vi "FPGA_Check_Pins_target.vi"() -> ()   [LabVIEW 2018]
uses:
  <vilib>/Platform/TimedLoop/XDataNode/timing_clust.ctl
  <vilib>/Platform/TimedLoop/XDataNode/nitl_modes.ctl
  <vilib>/Platform/TimedLoop/XDataNode/wakeup.ctl
  <vilib>/rvi/Emulation/niFpgaGetClockAttributes.vi
  <vilib>/rvi/Emulation/niFpgaSctlEmulationGetInTimedLoop.vi
  <vilib>/rvi/Emulation/niFpgaEmulationReportErrorSimple.vi
  <vilib>/rvi/eio/common/nirviEmuTemplateMethod_errors.vi
  <vilib>/rvi/Emulation/niFpgaCriticalErrorInLSC.vi
  <vilib>/rvi/Emulation/niFpgaProcessEmulError.vi
  <vilib>/eio/EIONode/EIONode.xnode
  <vilib>/Platform/TimedLoop/XDataNode/XDataNode.xnode
  <vilib>/Platform/TimedLoop/XDataNode/XDNodeRunTimeDep.lvlib
panel:
  out "Delay B to A":i16
  out "0 (B to A)":bool
  out "1 (B to A)":bool
  out "2 (B to A)":bool
  out "3 (B to A)":bool
  out "4 (B to A)":bool
  out "5 (B to A)":bool
  out "6 (B to A)":bool
  out "7 (B to A)":bool
  out "DDCA_PFI1_Read (B to A)":bool
  out "DDCA_PFI2_Read (B to A)":bool
  out "DDCA_PFI3_Read (B to A)":bool
  out "Number (B to A)":i16
  out "Delay 0.0 (B to A)":i16
  out "Delay 0.1 (B to A)":i16
  out "Delay 0.2 (B to A)":i16
  out "Delay 0.3 (B to A)":i16
  out "Delay 0.4 (B to A)":i16
  out "Delay 0.5 (B to A)":i16
  out "Delay 0.6 (B to A)":i16
  out "Delay 0.7 (B to A)":i16
  out "Delay 1.0 (B to A)":i16
  out "Delay 1.1 (B to A)":i16
  out "Delay 1.2 (B to A)":i16
  out "Delay 1.3 (B to A)":i16
  out "Delay 1.4 (B to A)":i16
  out "Delay 1.5 (B to A)":i16
  out "Delay 1.6 (B to A)":i16
  out "Delay 1.7 (B to A)":i16
  out "Delay PFI1 (B to A)":i16
  out "Delay PFI2 (B to A)":i16
  out "Delay PFI3 (B to A)":i16
  out "Delay 2.0 (B to A)":i16
  out "Delay 2.1 (B to A)":i16
  out "Delay 2.2 (B to A)":i16
  out "Delay 2.3 (B to A)":i16
  out "Delay 2.4 (B to A)":i16
  out "Delay 2.5 (B to A)":i16
  out "Delay 2.6 (B to A)":i16
  out "Delay 2.7 (B to A)":i16
  out "Read Port 0 A":u8 format="%b"
  out "Read Port 1 A":u8 format="%b"
  out "Read Port 2 A":u8 format="%b"
  out "DDCA_PFI1_Read 3":bool
  out "DDCA_PFI2_Read 3":bool
  out "DDCA_PFI3_Read 3":bool
  out "Delay A to B":i16
  out "DDCB_PFI3_Read (A to B)":bool
  out "DDCB_PFI2_Read (A to B)":bool
  out "DDCB_PFI1_Read (A to B)":bool
  out "Read Port 2 B":u8 format="%b"
  out "Read Port 1 B":u8 format="%b"
  out "Read Port 0 B":u8 format="%b"
  out "Delay 2.0":i16
  out "Delay 2.1":i16
  out "Delay 2.2":i16
  out "Delay 2.3":i16
  out "Delay 2.4":i16
  out "Delay 2.5":i16
  out "Delay 2.6":i16
  out "Delay 2.7":i16
  out "Delay PFI1":i16
  out "Delay PFI2":i16
  out "Delay PFI3":i16
  out "Delay 1.0":i16
  out "Delay 1.1":i16
  out "Delay 1.2":i16
  out "Delay 1.3":i16
  out "Delay 1.4":i16
  out "Delay 1.5":i16
  out "Delay 1.6":i16
  out "Delay 1.7":i16
  out "Delay 0.7":i16
  out "Delay 0.6":i16
  out "Delay 0.5":i16
  out "Delay 0.4":i16
  out "Delay 0.3":i16
  out "Delay 0.2":i16
  out "Delay 0.1":i16
  out "PFI 3  (A to B)":bool
  out "PFI 2  (A to B)":bool
  out "PFI 1  (A to B)":bool
  out "7":bool
  out "6":bool
  out "5":bool
  out "4":bool
  out "3":bool
  out "2":bool
  out "1":bool
  out "0":bool
  in  "Counter":i16
  out "Delay 0.0":i16
  out "Operation compl":bool
  in  "Write to PFI":u8
  in  "Cycle":bool
  in  "A to B/B to A":bool
  in  "Write to":u8 format="%b"
  in  "Source Freq":refnum<k21>="100 MHz Clock"
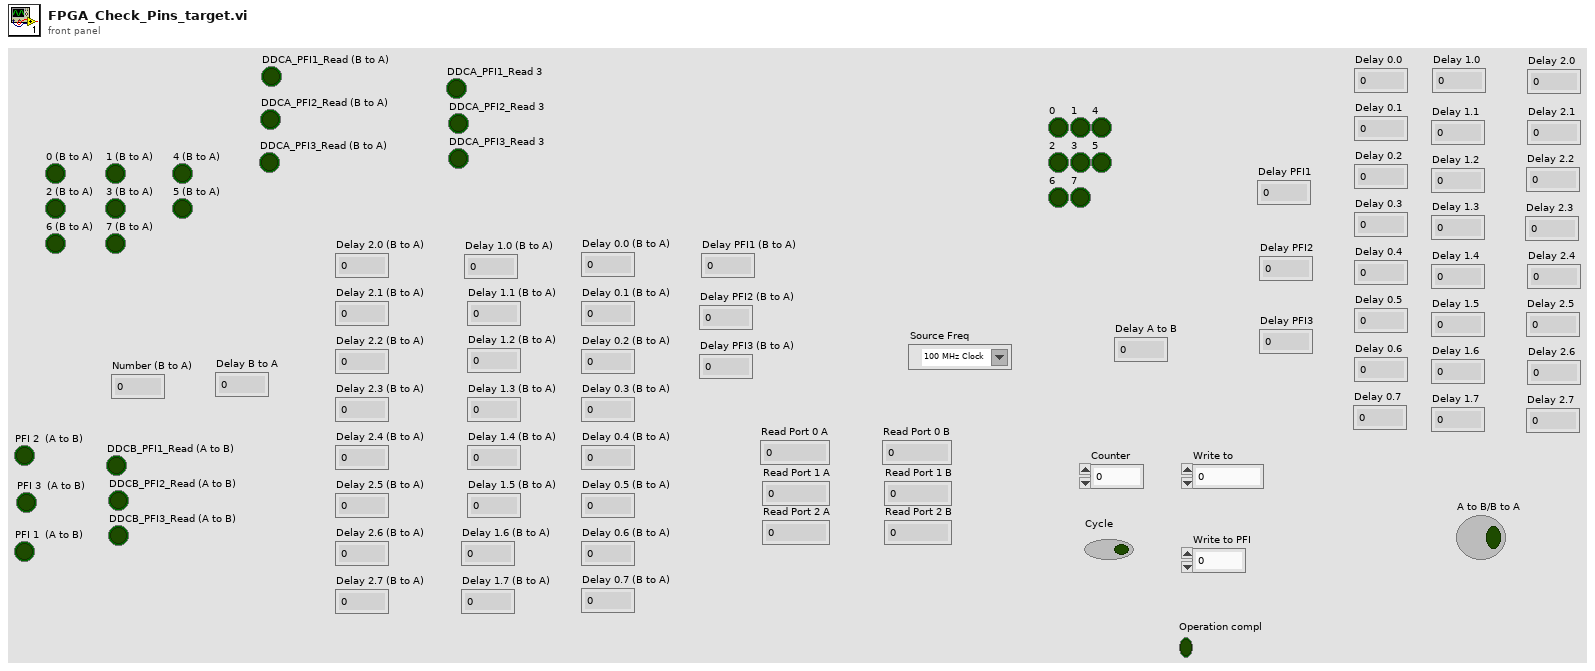
[diagram p1: front panel]
types:
  T1 = typedef "XDNodeRunTimeDep.lvlib/timing_clust.ctl" = cluster{"Expected End [f-1]":u64, "Actual End [f-1]":u64, "Finished Late? [f-1]":bool, "Expected End [i-1]":u64, "Actual End [i-1]":u64, "Finished Late? [i-1]":bool, "Expected Start [i]":u64, "Actual Start [i]":u64, "Expected Start [f]":u64, "Actual Start [f]":u64, "Source Name":string, "Structure Name":string, "Period":i64, "Deadline":i64, "Offset":i64, "Start":i64, "Priority":i32, "Timeout":i32, "Mode":T2, "Wakeup Reason":T3, "Error":errorcluster, "Source Type":string, "Secondary Source Type":string, "Global End Time":u64, "Global Start Time":u64, "Frame Duration":u64, "Iteration Duration":u64, "Assigned CPU":i32, "I/O Scan Engine Mode":u32}
  T2 = typedef "XDNodeRunTimeDep.lvlib/nitl_modes.ctl" = enum32{"No Change", "Process missed periods, maintain original phase", "Discard missed periods, maintain original phase", "Process missed periods, ignore original phase", "Discard missed periods, ignore original phase"}
  T3 = typedef "XDNodeRunTimeDep.lvlib/wakeup.ctl" = enum32{"Normal", "Aborted", "Asynchronous wakeup", "Timing source error", "Timed loop error", "Timeout"}
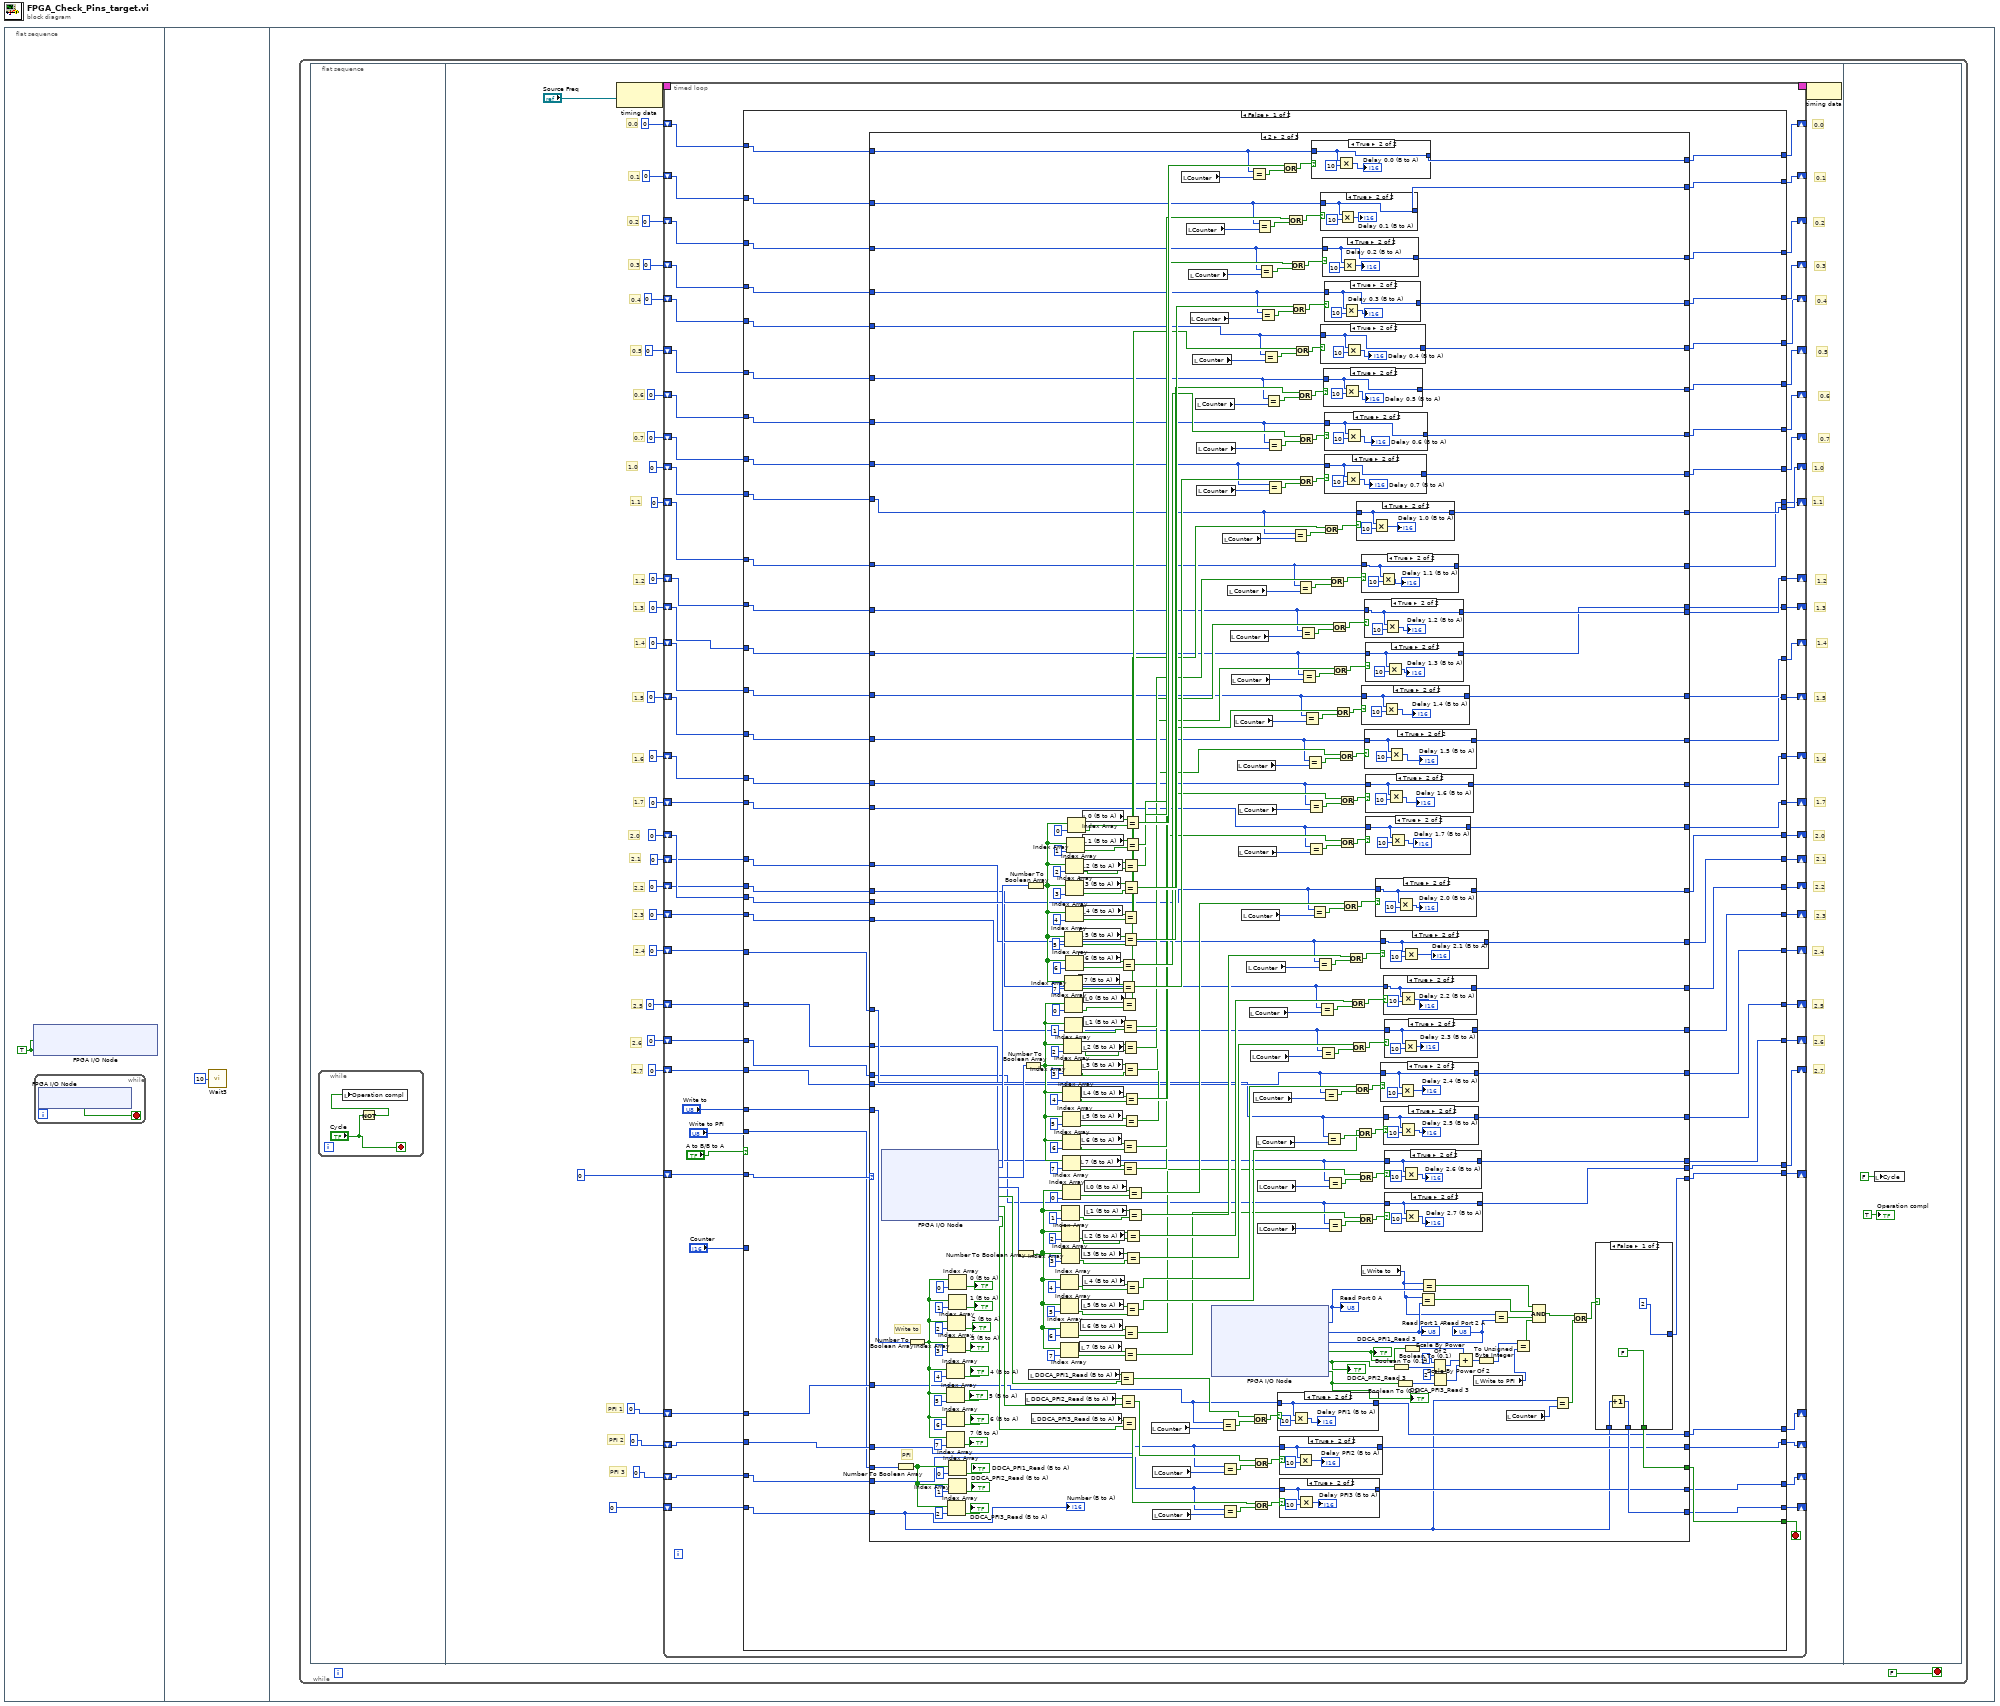
[diagram p0: block diagram]
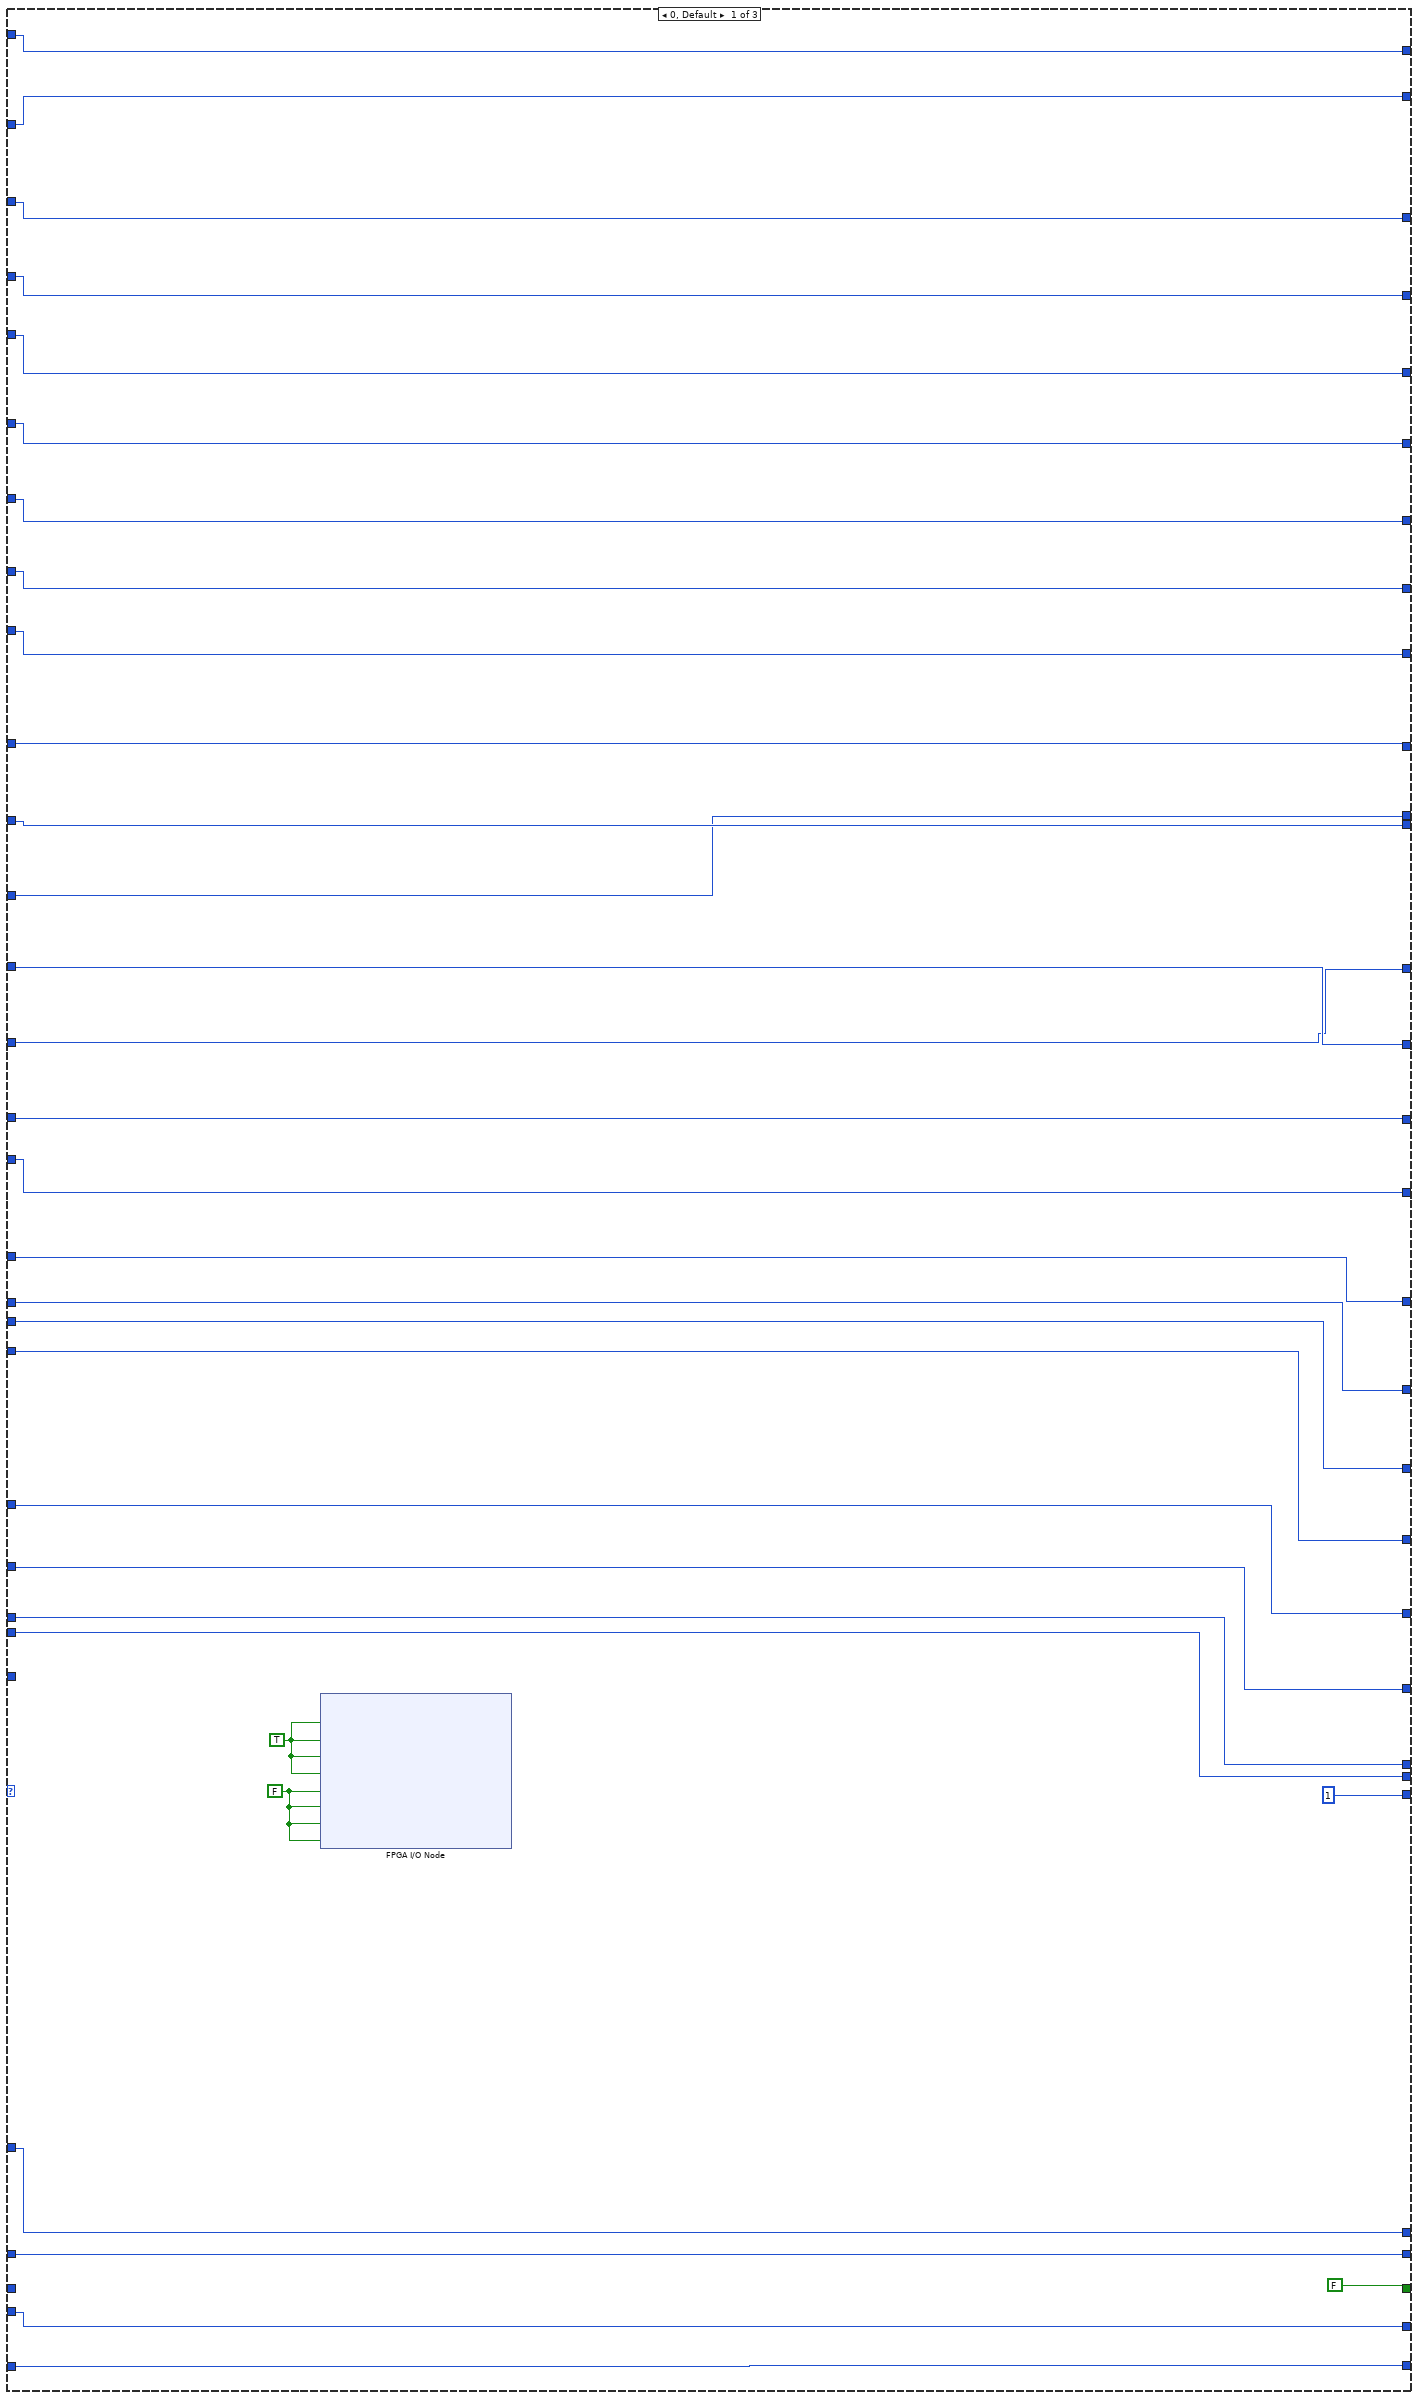
[diagram p2: hidden frame]
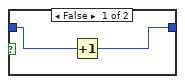
[diagram p3: hidden frame]
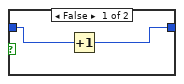
[diagram p4: hidden frame]
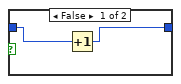
[diagram p5: hidden frame]
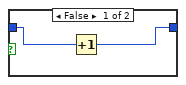
[diagram p6: hidden frame]
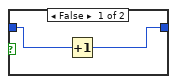
[diagram p7: hidden frame]
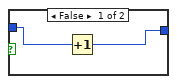
[diagram p8: hidden frame]
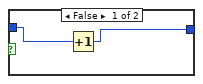
[diagram p9: hidden frame]
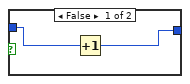
[diagram p10: hidden frame]
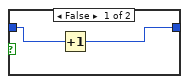
[diagram p11: hidden frame]
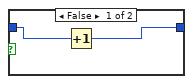
[diagram p12: hidden frame]
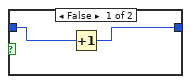
[diagram p13: hidden frame]
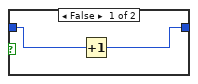
[diagram p14: hidden frame]
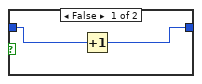
[diagram p15: hidden frame]
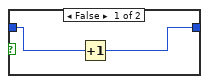
[diagram p16: hidden frame]
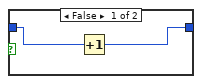
[diagram p17: hidden frame]
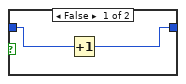
[diagram p18: hidden frame]
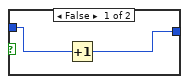
[diagram p19: hidden frame]
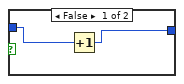
[diagram p20: hidden frame]
diagram:
  n1 = flat-sequence {
    frame #0 {
      w1 = TRUE ("IO Module\\DDCB_Supply_Select")
      n2 = xnode "FPGA I/O Node"("IO Module\\DDCB_Supply_Select"=w1, "IO Module\\DDCA_Supply_Select"=w1) -> ()  [unwired: 2 in, 2 out]
      n3 = while {
        stop <- w2 stop-if-true
        n4 = xnode "FPGA I/O Node"() -> ("IO Module IO Enabled"=w2:bool)  [unwired: 1 in, 1 out]
      }
    }
    frame #1 {
      n5 = call "Wait3"("Count(mSec)"=u8 10) -> ()  [unwired: 1 out]
    }
    frame #2 {
      n6 = while {
        stop <- FALSE stop-if-true
        n7 = flat-sequence {
          frame #0 {
            n8 = while {
              stop <- "Cycle" stop-if-true
              n9 = Not(x="Cycle") -> (.not. x?=w5:bool)
              n10 = local write "Operation compl"(w5) -> ()
            }
          }
          frame #1 {
            # "2.7"
            # "2.6"
            # "2.5"
            # "2.4"
            # "2.3"
            # "2.2"
            # "2.1"
            # "2.0"
            # "1.0"
            # "1.7"
            # "1.6"
            # "1.5"
            # "1.4"
            # "1.3"
            # "1.2"
            # "1.1"
            # "0.7"
            # "0.6"
            # "0.5"
            # "0.4"
            # "0.3"
            # "0.2"
            # "0.1"
            # "0.0"
            # "2.7"
            # "2.6"
            # "2.5"
            # "2.4"
            # "2.3"
            # "2.2"
            # "2.1"
            # "2.0"
            # "PFI 3"
            # "PFI 2"
            # "PFI 1"
            # "1.7"
            # "1.6"
            # "1.5"
            # "1.4"
            # "1.3"
            # "1.2"
            # "1.1"
            # "1.0"
            # "0.7"
            # "0.6"
            # "0.5"
            # "0.4"
            # "0.3"
            # "0.2"
            # "0.1"
            # "0.0"
            n11 = node-c288("Source Freq") -> (w38:T1)
            n12 = timed-loop {
              timing: w38 -> [_]
              timing-out: [_] -> w37
              shift-right: [w100] -> _
              shift-left: i16 0 -> [w101]
              shift-right: [w95] -> _
              shift-left: i16 0 -> [w94]
              shift-right: [w92] -> _
              shift-left: i16 0 -> [w91]
              shift-right: [w89] -> _
              shift-left: i16 0 -> [w90]
              shift-right: [w87] -> _
              shift-left: i16 0 -> [w88]
              shift-right: [w81] -> _
              shift-left: i16 0 -> [w86]
              shift-right: [w80] -> _
              shift-left: i16 0 -> [w85]
              shift-right: [w79] -> _
              shift-left: i16 0 -> [w84]
              shift-right: [w78] -> _
              shift-left: i16 0 -> [w83]
              shift-right: [w77] -> _
              shift-left: i16 0 -> [w82]
              shift-right: [w71] -> _
              shift-left: i16 0 -> [w76]
              shift-right: [w72] -> _
              shift-left: i16 0 -> [w75]
              shift-right: [w73] -> _
              shift-left: i16 0 -> [w74]
              shift-right: [w54] -> _
              shift-left: i16 0 -> [w70]
              shift-right: [w53] -> _
              shift-left: i16 0 -> [w69]
              shift-right: [w52] -> _
              shift-left: i16 0 -> [w68]
              shift-right: [w51] -> _
              shift-left: i16 0 -> [w67]
              shift-right: [w50] -> _
              shift-left: i16 0 -> [w66]
              shift-right: [w49] -> _
              shift-left: i16 0 -> [w65]
              shift-right: [w48] -> _
              shift-left: i16 0 -> [w64]
              shift-right: [w47] -> _
              shift-left: i16 0 -> [w63]
              shift-right: [w46] -> _
              shift-left: i16 0 -> [w62]
              shift-right: [w45] -> _
              shift-left: i16 0 -> [w61]
              shift-right: [w44] -> _
              shift-left: i16 0 -> [w60]
              shift-right: [w43] -> _
              shift-left: i16 0 -> [w59]
              shift-right: [w42] -> _
              shift-left: i16 0 -> [w58]
              shift-right: [w41] -> _
              shift-left: i16 0 -> [w57]
              shift-right: [w40] -> _
              shift-left: i16 0 -> [w56]
              shift-right: [w39] -> _
              shift-left: i16 0 -> [w55]
              stop <- w99 stop-if-true
              n13 = case shown="False" "A to B/B to A" {
                tunnel: w101 -> [w160 w738]
                tunnel: [w108 w737] -> w100
                tunnel: [w105 w736] -> w99
                tunnel: "Write to PFI" -> [w157 w678]
                tunnel: "Write to" -> [w156 w677]
                tunnel: [w104 w735] -> w95
                tunnel: w94 -> [w162 w734]
                tunnel: "Counter" -> [_ w733]
                tunnel: [w155 w732] -> w92
                tunnel: w91 -> [w154 w731]
                tunnel: w90 -> [w153 w730]
                tunnel: [w130 w729] -> w89
                tunnel: w88 -> [w152 w728]
                tunnel: [w129 w727] -> w87
                tunnel: w86 -> [w151 w726]
                tunnel: w85 -> [w150 w725]
                tunnel: w84 -> [w149 w724]
                tunnel: w83 -> [w148 w723]
                tunnel: w82 -> [w147 w722]
                tunnel: [w128 w721] -> w81
                tunnel: [w127 w720] -> w80
                tunnel: [w126 w719] -> w79
                tunnel: [w125 w718] -> w78
                tunnel: [w124 w717] -> w77
                tunnel: w76 -> [w159 w716]
                tunnel: w75 -> [w158 w715]
                tunnel: w74 -> [w161 w714]
                tunnel: [w103 w713] -> w73
                tunnel: [w102 w712] -> w72
                tunnel: [w106 w711] -> w71
                tunnel: w70 -> [w146 w710]
                tunnel: w69 -> [w145 w709]
                tunnel: w68 -> [w144 w708]
                tunnel: w67 -> [w143 w707]
                tunnel: w66 -> [w142 w706]
                tunnel: w65 -> [w141 w705]
                tunnel: w64 -> [w140 w704]
                tunnel: w63 -> [w139 w703]
                tunnel: w62 -> [w136 w702]
                tunnel: w61 -> [w138 w701]
                tunnel: w60 -> [w137 w700]
                tunnel: w59 -> [w135 w699]
                tunnel: w58 -> [w134 w698]
                tunnel: w57 -> [w133 w697]
                tunnel: w56 -> [w132 w696]
                tunnel: w55 -> [w131 w695]
                tunnel: [w123 w694] -> w54
                tunnel: [w122 w693] -> w53
                tunnel: [w121 w692] -> w52
                tunnel: [w120 w691] -> w51
                tunnel: [w119 w690] -> w50
                tunnel: [w118 w689] -> w49
                tunnel: [w117 w688] -> w48
                tunnel: [w116 w687] -> w47
                tunnel: [w115 w686] -> w46
                tunnel: [w114 w685] -> w45
                tunnel: [w113 w684] -> w44
                tunnel: [w112 w683] -> w43
                tunnel: [w111 w682] -> w42
                tunnel: [w110 w681] -> w41
                tunnel: [w109 w680] -> w40
                tunnel: [w107 w679] -> w39
                frame False {
                  n14 = case shown="2" w160 {
                    tunnel: [i16 1 w495 i16 2] -> w108
                    tunnel: [FALSE w494 FALSE] -> w105
                    tunnel: [w192 w249 w667] -> w104
                    tunnel: w162 -> [w192 w195 w667]
                    tunnel: w156 -> [_ w493 w638]
                    tunnel: w157 -> [_ w483 w639]
                    tunnel: [w189 w250 w666] -> w155
                    tunnel: w154 -> [w189 w248 w666]
                    tunnel: w153 -> [w188 w247 w665]
                    tunnel: [w188 w246 w665] -> w130
                    tunnel: w152 -> [w187 w245 w664]
                    tunnel: [w187 w244 w664] -> w129
                    tunnel: w151 -> [w186 w243 w663]
                    tunnel: w150 -> [w185 w242 w662]
                    tunnel: w149 -> [w184 w241 w661]
                    tunnel: w148 -> [w183 w240 w660]
                    tunnel: w147 -> [w182 w239 w659]
                    tunnel: [w186 w238 w663] -> w128
                    tunnel: [w185 w237 w662] -> w127
                    tunnel: [w184 w236 w661] -> w126
                    tunnel: [w183 w235 w660] -> w125
                    tunnel: [w182 w234 w659] -> w124
                    tunnel: w159 -> [w163 w233 w640]
                    tunnel: w158 -> [w164 w232 w641]
                    tunnel: w161 -> [w165 w231 w642]
                    tunnel: [w165 w230 w642] -> w103
                    tunnel: [w164 w229 w641] -> w102
                    tunnel: [w163 w228 w640] -> w106
                    tunnel: w146 -> [w181 w227 w658]
                    tunnel: w145 -> [w180 w226 w657]
                    tunnel: w144 -> [w179 w225 w656]
                    tunnel: w143 -> [w178 w224 w655]
                    tunnel: w142 -> [w177 w223 w654]
                    tunnel: w141 -> [w176 w222 w653]
                    tunnel: w140 -> [w175 w221 w652]
                    tunnel: w139 -> [w174 w220 w651]
                    tunnel: w136 -> [w171 w219 w650]
                    tunnel: w138 -> [w173 w218 w649]
                    tunnel: w137 -> [w172 w217 w648]
                    tunnel: w135 -> [w170 w216 w647]
                    tunnel: w131 -> [w166 w215 w643]
                    tunnel: w134 -> [w169 w214 w646]
                    tunnel: w133 -> [w168 w213 w645]
                    tunnel: w132 -> [w167 w212 w644]
                    tunnel: [w181 w211 w658] -> w123
                    tunnel: [w180 w210 w657] -> w122
                    tunnel: [w179 w209 w656] -> w121
                    tunnel: [w178 w208 w655] -> w120
                    tunnel: [w176 w207 w654] -> w119
                    tunnel: [w177 w206 w653] -> w118
                    tunnel: [w175 w205 w652] -> w117
                    tunnel: [w174 w204 w651] -> w116
                    tunnel: [w173 w203 w650] -> w115
                    tunnel: [w172 w202 w649] -> w114
                    tunnel: [w171 w201 w648] -> w113
                    tunnel: [w170 w200 w647] -> w112
                    tunnel: [w169 w199 w646] -> w111
                    tunnel: [w168 w198 w645] -> w110
                    tunnel: [w167 w197 w644] -> w109
                    tunnel: [w166 w196 w643] -> w107
                    frame 0, Default {
                      w190 = FALSE ("IO Module\\DDCB_Port0_WE")
                      w194 = TRUE
                      n15 = xnode "FPGA I/O Node"("IO Module\\DDCB_Port0_WE"=w194, "IO Module\\DDCB_Port1_WE"=w194, "IO Module\\DDCB_Port2_WE"=w194, "IO Module\\DDCB_PFI_WE"=w194, "IO Module\\DDCA_Port0_WE"=w190, "IO Module\\DDCA_Port1_WE"=w190, "IO Module\\DDCA_Port2_WE"=w190, "IO Module\\DDCA_PFI_WE"=w190) -> ()  [unwired: 8 in, 8 out]
                    }
                    frame 2 {
                      # "Write to"
                      # "PFI"
                      n16 = xnode "FPGA I/O Node"() -> ("IO Module\\DDCA_Port0_Read"=w469:u8, "IO Module\\DDCA_Port1_Read"=w459:u8, "IO Module\\DDCA_Port2_Read"=w449:u8, "IO Module\\DDCA_PFI1_Read"=w386:bool, "IO Module\\DDCA_PFI2_Read"=w385:bool, "IO Module\\DDCA_PFI3_Read"=w384:bool)  [unwired: 6 in, 6 out]
                      n17 = Number To Boolean Array(number=w483) -> (Boolean array=w479:bool[])
                      n18 = Number To Boolean Array(number=w493) -> (Boolean array=w492:bool[])
                      n19 = Index Array(array=w492, index=5) -> (element=→"5 (B to A)":bool)
                      n20 = Index Array(array=w492, index=7) -> (element=→"7 (B to A)":bool)
                      n21 = Index Array(array=w492, index=4) -> (element=→"4 (B to A)":bool)
                      n22 = Index Array(array=w492, index=6) -> (element=→"6 (B to A)":bool)
                      n23 = Index Array(array=w492, index=2) -> (element=→"2 (B to A)":bool)
                      n24 = Index Array(array=w492, index=3) -> (element=→"3 (B to A)":bool)
                      n25 = Index Array(array=w479, index=2) -> (element=→"DDCA_PFI3_Read (B to A)":bool)
                      n26 = Index Array(array=w492, index=1) -> (element=→"1 (B to A)":bool)
                      n27 = Index Array(array=w479, index=1) -> (element=→"DDCA_PFI2_Read (B to A)":bool)
                      n28 = Index Array(array=w492, index=0) -> (element=→"0 (B to A)":bool)
                      n29 = Index Array(array=w479, index=0) -> (element=→"DDCA_PFI1_Read (B to A)":bool)
                      n30 = Number To Boolean Array(number=w449) -> (Boolean array=w450:bool[])
                      n31 = Number To Boolean Array(number=w459) -> (Boolean array=w468:bool[])
                      n32 = local read "DDCA_PFI2_Read (B to A)"() -> (w388:bool)
                      n33 = Number To Boolean Array(number=w469) -> (Boolean array=w470:bool[])
                      n34 = local read "DDCA_PFI1_Read (B to A)"() -> (w389:bool)
                      n35 = local read "DDCA_PFI3_Read (B to A)"() -> (w387:bool)
                      n36 = Index Array(array=w450, index=5) -> (element=w392:bool)
                      n37 = Index Array(array=w450, index=7) -> (element=w390:bool)
                      n38 = Index Array(array=w450, index=4) -> (element=w393:bool)
                      n39 = Index Array(array=w450, index=6) -> (element=w391:bool)
                      n40 = Index Array(array=w450, index=2) -> (element=w395:bool)
                      n41 = Index Array(array=w450, index=3) -> (element=w394:bool)
                      n42 = Index Array(array=w450, index=1) -> (element=w396:bool)
                      n43 = Index Array(array=w468, index=5) -> (element=w408:bool)
                      n44 = Index Array(array=w468, index=7) -> (element=w406:bool)
                      n45 = Index Array(array=w450, index=0) -> (element=w397:bool)
                      n46 = Index Array(array=w468, index=4) -> (element=w409:bool)
                      n47 = Index Array(array=w468, index=6) -> (element=w407:bool)
                      n48 = Index Array(array=w468, index=2) -> (element=w411:bool)
                      n49 = Index Array(array=w468, index=3) -> (element=w410:bool)
                      n50 = Index Array(array=w468, index=1) -> (element=w412:bool)
                      n51 = Index Array(array=w470, index=5) -> (element=w426:bool)
                      n52 = Index Array(array=w470, index=7) -> (element=w422:bool)
                      n53 = Index Array(array=w468, index=0) -> (element=w413:bool)
                      n54 = Index Array(array=w470, index=4) -> (element=w428:bool)
                      n55 = Index Array(array=w470, index=6) -> (element=w424:bool)
                      n56 = Index Array(array=w470, index=2) -> (element=w432:bool)
                      n57 = Index Array(array=w470, index=3) -> (element=w430:bool)
                      n58 = Index Array(array=w470, index=1) -> (element=w434:bool)
                      n59 = Index Array(array=w470, index=0) -> (element=w437:bool)
                      n60 = local read "7 (B to A)"() -> (w423:bool)
                      n61 = local read "6 (B to A)"() -> (w425:bool)
                      n62 = local read "3 (B to A)"() -> (w431:bool)
                      n63 = local read "5 (B to A)"() -> (w427:bool)
                      n64 = local read "7 (B to A)"() -> (w421:bool)
                      n65 = local read "6 (B to A)"() -> (w420:bool)
                      n66 = local read "7 (B to A)"() -> (w398:bool)
                      n67 = local read "2 (B to A)"() -> (w433:bool)
                      n68 = local read "4 (B to A)"() -> (w429:bool)
                      n69 = local read "3 (B to A)"() -> (w417:bool)
                      n70 = local read "5 (B to A)"() -> (w419:bool)
                      n71 = local read "6 (B to A)"() -> (w399:bool)
                      n72 = local read "2 (B to A)"() -> (w416:bool)
                      n73 = local read "4 (B to A)"() -> (w418:bool)
                      n74 = local read "3 (B to A)"() -> (w402:bool)
                      n75 = local read "5 (B to A)"() -> (w400:bool)
                      n76 = local read "0 (B to A)"() -> (w436:bool)
                      n77 = local read "1 (B to A)"() -> (w435:bool)
                      n78 = local read "2 (B to A)"() -> (w403:bool)
                      n79 = local read "4 (B to A)"() -> (w401:bool)
                      n80 = local read "0 (B to A)"() -> (w414:bool)
                      n81 = local read "1 (B to A)"() -> (w415:bool)
                      n82 = local read "0 (B to A)"() -> (w405:bool)
                      n83 = local read "1 (B to A)"() -> (w404:bool)
                      n84 = Equal?(x=w389, y=w386) -> (x = y?=w309:bool)
                      n85 = Equal?(x=w388, y=w385) -> (x = y?=w308:bool)
                      n86 = Equal?(x=w425, y=w424) -> (x = y?=w353:bool)
                      n87 = Equal?(x=w423, y=w422) -> (x = y?=w352:bool)
                      n88 = Equal?(x=w414, y=w413) -> (x = y?=w326:bool)
                      n89 = Equal?(x=w387, y=w384) -> (x = y?=w307:bool)
                      n90 = Equal?(x=w415, y=w412) -> (x = y?=w325:bool)
                      n91 = Equal?(x=w420, y=w407) -> (x = y?=w320:bool)
                      n92 = Equal?(x=w421, y=w406) -> (x = y?=w319:bool)
                      n93 = Equal?(x=w429, y=w428) -> (x = y?=w364:bool)
                      n94 = Equal?(x=w427, y=w426) -> (x = y?=w354:bool)
                      n95 = Equal?(x=w416, y=w411) -> (x = y?=w324:bool)
                      n96 = Equal?(x=w398, y=w390) -> (x = y?=w275:bool)
                      n97 = Equal?(x=w433, y=w432) -> (x = y?=w372:bool)
                      n98 = Equal?(x=w431, y=w430) -> (x = y?=w368:bool)
                      n99 = Equal?(x=w417, y=w410) -> (x = y?=w323:bool)
                      n100 = Equal?(x=w399, y=w391) -> (x = y?=w276:bool)
                      n101 = Equal?(x=w418, y=w409) -> (x = y?=w322:bool)
                      n102 = Equal?(x=w419, y=w408) -> (x = y?=w321:bool)
                      n103 = Equal?(x=w436, y=w437) -> (x = y?=w383:bool)
                      n104 = Equal?(x=w435, y=w434) -> (x = y?=w376:bool)
                      n105 = Equal?(x=w401, y=w393) -> (x = y?=w278:bool)
                      n106 = Equal?(x=w400, y=w392) -> (x = y?=w277:bool)
                      n107 = Equal?(x=w403, y=w395) -> (x = y?=w280:bool)
                      n108 = Equal?(x=w402, y=w394) -> (x = y?=w279:bool)
                      n109 = Equal?(x=w405, y=w397) -> (x = y?=w282:bool)
                      n110 = Equal?(x=w404, y=w396) -> (x = y?=w281:bool)
                      n111 = local read "Counter"() -> (w316:i16)
                      n112 = local read "Counter"() -> (w315:i16)
                      n113 = local read "Counter"() -> (w310:i16)
                      n114 = local read "Counter"() -> (w382:i16)
                      n115 = local read "Counter"() -> (w377:i16)
                      n116 = local read "Counter"() -> (w375:i16)
                      n117 = local read "Counter"() -> (w369:i16)
                      n118 = local read "Counter"() -> (w367:i16)
                      n119 = local read "Counter"() -> (w361:i16)
                      n120 = local read "Counter"() -> (w360:i16)
                      n121 = local read "Counter"() -> (w355:i16)
                      n122 = xnode "FPGA I/O Node"() -> ("IO Module\\DDCA_Port0_Read"=w274:u8, "IO Module\\DDCA_Port1_Read"=w273:u8, "IO Module\\DDCA_Port2_Read"=w272:u8, "IO Module\\DDCA_PFI1_Read"=w271:bool, "IO Module\\DDCA_PFI2_Read"=w269:bool, "IO Module\\DDCA_PFI3_Read"=w270:bool)  [unwired: 6 in, 6 out]
                      "Read Port 0 A" <- w274
                      "Read Port 1 A" <- w273
                      "Read Port 2 A" <- w272
                      "DDCA_PFI1_Read 3" <- w271
                      "DDCA_PFI2_Read 3" <- w269
                      "DDCA_PFI3_Read 3" <- w270
                      n123 = Equal?(x=w233, y=w316) -> (x = y?=w317:bool)
                      n124 = Equal?(x=w232, y=w315) -> (x = y?=w314:bool)
                      n125 = Equal?(x=w231, y=w310) -> (x = y?=w311:bool)
                      n126 = local read "Counter"() -> (w327:i16)
                      n127 = local read "Counter"() -> (w332:i16)
                      n128 = local read "Counter"() -> (w333:i16)
                      n129 = local read "Counter"() -> (w338:i16)
                      n130 = local read "Counter"() -> (w339:i16)
                      n131 = local read "Counter"() -> (w344:i16)
                      n132 = local read "Counter"() -> (w345:i16)
                      n133 = local read "Counter"() -> (w350:i16)
                      n134 = local read "Counter"() -> (w306:i16)
                      n135 = local read "Counter"() -> (w301:i16)
                      n136 = local read "Counter"() -> (w300:i16)
                      n137 = Equal?(x=w248, y=w382) -> (x = y?=w381:bool)
                      n138 = local read "Counter"() -> (w295:i16)
                      n139 = Or(x=w309, y=w317) -> (x .or. y?=w318:bool)
                      n140 = Or(x=w308, y=w314) -> (x .or. y?=w313:bool)
                      n141 = Or(x=w307, y=w311) -> (x .or. y?=w312:bool)
                      n142 = local read "Counter"() -> (w294:i16)
                      n143 = Equal?(x=w247, y=w377) -> (x = y?=w378:bool)
                      n144 = local read "Counter"() -> (w289:i16)
                      n145 = local read "Counter"() -> (w288:i16)
                      n146 = local read "Counter"() -> (w283:i16)
                      n147 = Equal?(x=w245, y=w375) -> (x = y?=w374:bool)
                      n148 = Equal?(x=w243, y=w369) -> (x = y?=w370:bool)
                      n149 = Equal?(x=w242, y=w367) -> (x = y?=w366:bool)
                      n150 = Equal?(x=w241, y=w361) -> (x = y?=w362:bool)
                      n151 = Equal?(x=w240, y=w360) -> (x = y?=w359:bool)
                      n152 = Equal?(x=w239, y=w355) -> (x = y?=w356:bool)
                      n153 = case shown="True" w318 {
                        tunnel: w233 -> [w547 w548]
                        tunnel: [w546 w548] -> w228
                        frame False {
                          n154 = Increment(x=w547) -> (x+1=w546:i16)
                        }
                        frame True {
                          n155 = Multiply(x=w548, y=i16 10) -> (x*y=→"Delay PFI1 (B to A)":i16)
                        }
                      }
                      n156 = case shown="True" w313 {
                        tunnel: w232 -> [w542 w544]
                        tunnel: [w541 w544] -> w229
                        frame False {
                          n157 = Increment(x=w542) -> (x+1=w541:i16)
                        }
                        frame True {
                          n158 = Multiply(x=w544, y=i16 10) -> (x*y=→"Delay PFI2 (B to A)":i16)
                        }
                      }
                      n159 = case shown="True" w312 {
                        tunnel: w231 -> [w537 w539]
                        tunnel: [w536 w539] -> w230
                        frame False {
                          n160 = Increment(x=w537) -> (x+1=w536:i16)
                        }
                        frame True {
                          n161 = Multiply(x=w539, y=i16 10) -> (x*y=→"Delay PFI3 (B to A)":i16)
                        }
                      }
                      n162 = Or(x=w383, y=w381) -> (x .or. y?=w380:bool)
                      n163 = Or(x=w376, y=w378) -> (x .or. y?=w379:bool)
                      n164 = Or(x=w372, y=w374) -> (x .or. y?=w373:bool)
                      n165 = Or(x=w368, y=w370) -> (x .or. y?=w371:bool)
                      n166 = Equal?(x=w227, y=w327) -> (x = y?=w328:bool)
                      n167 = Or(x=w364, y=w366) -> (x .or. y?=w365:bool)
                      n168 = Or(x=w354, y=w362) -> (x .or. y?=w363:bool)
                      n169 = Equal?(x=w226, y=w332) -> (x = y?=w331:bool)
                      n170 = Or(x=w353, y=w359) -> (x .or. y?=w358:bool)
                      n171 = Or(x=w352, y=w356) -> (x .or. y?=w357:bool)
                      n172 = Equal?(x=w225, y=w333) -> (x = y?=w334:bool)
                      n173 = Equal?(x=w224, y=w338) -> (x = y?=w337:bool)
                      n174 = Equal?(x=w223, y=w339) -> (x = y?=w340:bool)
                      n175 = Equal?(x=w222, y=w344) -> (x = y?=w343:bool)
                      n176 = Equal?(x=w221, y=w345) -> (x = y?=w346:bool)
                      n177 = Equal?(x=w220, y=w350) -> (x = y?=w349:bool)
                      n178 = Equal?(x=w219, y=w306) -> (x = y?=w305:bool)
                      n179 = case shown="True" w380 {
                        tunnel: w248 -> [w626 w630]
                        tunnel: [w627 w630] -> w250
                        frame False {
                          n180 = Increment(x=w626) -> (x+1=w627:i16)
                        }
                        frame True {
                          n181 = Multiply(x=w630, y=i16 10) -> (x*y=→"Delay 0.0 (B to A)":i16)
                        }
                      }
                      n182 = Equal?(x=w218, y=w301) -> (x = y?=w302:bool)
                      n183 = Equal?(x=w217, y=w300) -> (x = y?=w299:bool)
                      n184 = Equal?(x=w216, y=w295) -> (x = y?=w296:bool)
                      n185 = case shown="True" w379 {
                        tunnel: w247 -> [w622 w623]
                        tunnel: [w621 w623] -> w246
                        frame False {
                          n186 = Increment(x=w622) -> (x+1=w621:i16)
                        }
                        frame True {
                          n187 = Multiply(x=w623, y=i16 10) -> (x*y=→"Delay 0.1 (B to A)":i16)
                        }
                      }
                      n188 = case shown="True" w365 {
                        tunnel: w242 -> [w607 w609]
                        tunnel: [w606 w609] -> w237
                        frame False {
                          n189 = Increment(x=w607) -> (x+1=w606:i16)
                        }
                        frame True {
                          n190 = Multiply(x=w609, y=i16 10) -> (x*y=→"Delay 0.4 (B to A)":i16)
                        }
                      }
                      n191 = Equal?(x=w215, y=w294) -> (x = y?=w293:bool)
                      n192 = case shown="True" w373 {
                        tunnel: w245 -> [w617 w619]
                        tunnel: [w616 w619] -> w244
                        frame False {
                          n193 = Increment(x=w617) -> (x+1=w616:i16)
                        }
                        frame True {
                          n194 = Multiply(x=w619, y=i16 10) -> (x*y=→"Delay 0.2 (B to A)":i16)
                        }
                      }
                      n195 = Or(x=w326, y=w328) -> (x .or. y?=w329:bool)
                      n196 = case shown="True" w363 {
                        tunnel: w241 -> [w602 w603]
                        tunnel: [w601 w603] -> w236
                        frame False {
                          n197 = Increment(x=w602) -> (x+1=w601:i16)
                        }
                        frame True {
                          n198 = Multiply(x=w603, y=i16 10) -> (x*y=→"Delay 0.5 (B to A)":i16)
                        }
                      }
                      n199 = case shown="True" w371 {
                        tunnel: w243 -> [w612 w613]
                        tunnel: [w611 w613] -> w238
                        frame False {
                          n200 = Increment(x=w612) -> (x+1=w611:i16)
                        }
                        frame True {
                          n201 = Multiply(x=w613, y=i16 10) -> (x*y=→"Delay 0.3 (B to A)":i16)
                        }
                      }
                      n202 = case shown="True" w358 {
                        tunnel: w240 -> [w597 w599]
                        tunnel: [w596 w599] -> w235
                        frame False {
                          n203 = Increment(x=w597) -> (x+1=w596:i16)
                        }
                        frame True {
                          n204 = Multiply(x=w599, y=i16 10) -> (x*y=→"Delay 0.6 (B to A)":i16)
                        }
                      }
                      n205 = case shown="True" w357 {
                        tunnel: w239 -> [w592 w593]
                        tunnel: [w591 w593] -> w234
                        frame False {
                          n206 = Increment(x=w592) -> (x+1=w591:i16)
                        }
                        frame True {
                          n207 = Multiply(x=w593, y=i16 10) -> (x*y=→"Delay 0.7 (B to A)":i16)
                        }
                      }
                      n208 = Equal?(x=w214, y=w289) -> (x = y?=w290:bool)
                      n209 = Equal?(x=w213, y=w288) -> (x = y?=w287:bool)
                      n210 = Equal?(x=w212, y=w283) -> (x = y?=w284:bool)
                      n211 = Or(x=w325, y=w331) -> (x .or. y?=w330:bool)
                      n212 = Or(x=w324, y=w334) -> (x .or. y?=w335:bool)
                      n213 = Or(x=w323, y=w337) -> (x .or. y?=w336:bool)
                      n214 = Or(x=w322, y=w340) -> (x .or. y?=w341:bool)
                      n215 = Or(x=w321, y=w343) -> (x .or. y?=w342:bool)
                      n216 = Or(x=w320, y=w346) -> (x .or. y?=w347:bool)
                      n217 = Or(x=w319, y=w349) -> (x .or. y?=w348:bool)
                      n218 = Or(x=w282, y=w305) -> (x .or. y?=w304:bool)
                      n219 = Or(x=w281, y=w302) -> (x .or. y?=w303:bool)
                      n220 = Or(x=w280, y=w299) -> (x .or. y?=w298:bool)
                      n221 = Or(x=w279, y=w296) -> (x .or. y?=w297:bool)
                      n222 = Or(x=w278, y=w293) -> (x .or. y?=w292:bool)
                      n223 = case shown="True" w329 {
                        tunnel: w227 -> [w587 w589]
                        tunnel: [w586 w589] -> w211
                        frame False {
                          n224 = Increment(x=w587) -> (x+1=w586:i16)
                        }
                        frame True {
                          n225 = Multiply(x=w589, y=i16 10) -> (x*y=→"Delay 1.0 (B to A)":i16)
                        }
                      }
                      n226 = Or(x=w277, y=w290) -> (x .or. y?=w291:bool)
                      n227 = Or(x=w276, y=w287) -> (x .or. y?=w286:bool)
                      n228 = Or(x=w275, y=w284) -> (x .or. y?=w285:bool)
                      n229 = local read "Write to"() -> (w260:u8)
                      n230 = case shown="True" w330 {
                        tunnel: w226 -> [w582 w584]
                        tunnel: [w581 w584] -> w210
                        frame False {
                          n231 = Increment(x=w582) -> (x+1=w581:i16)
                        }
                        frame True {
                          n232 = Multiply(x=w584, y=i16 10) -> (x*y=→"Delay 1.1 (B to A)":i16)
                        }
                      }
                      n233 = case shown="True" w341 {
                        tunnel: w223 -> [w567 w569]
                        tunnel: [w566 w569] -> w207
                        frame False {
                          n234 = Increment(x=w567) -> (x+1=w566:i16)
                        }
                        frame True {
                          n235 = Multiply(x=w569, y=i16 10) -> (x*y=→"Delay 1.4 (B to A)":i16)
                        }
                      }
                      n236 = case shown="True" w335 {
                        tunnel: w225 -> [w577 w578]
                        tunnel: [w576 w578] -> w209
                        frame False {
                          n237 = Increment(x=w577) -> (x+1=w576:i16)
                        }
                        frame True {
                          n238 = Multiply(x=w578, y=i16 10) -> (x*y=→"Delay 1.2 (B to A)":i16)
                        }
                      }
                      n239 = case shown="True" w342 {
                        tunnel: w222 -> [w562 w564]
                        tunnel: [w561 w564] -> w206
                        frame False {
                          n240 = Increment(x=w562) -> (x+1=w561:i16)
                        }
                        frame True {
                          n241 = Multiply(x=w564, y=i16 10) -> (x*y=→"Delay 1.5 (B to A)":i16)
                        }
                      }
                      n242 = case shown="True" w336 {
                        tunnel: w224 -> [w572 w573]
                        tunnel: [w571 w573] -> w208
                        frame False {
                          n243 = Increment(x=w572) -> (x+1=w571:i16)
                        }
                        frame True {
                          n244 = Multiply(x=w573, y=i16 10) -> (x*y=→"Delay 1.3 (B to A)":i16)
                        }
                      }
                      n245 = case shown="True" w347 {
                        tunnel: w221 -> [w557 w558]
                        tunnel: [w556 w558] -> w205
                        frame False {
                          n246 = Increment(x=w557) -> (x+1=w556:i16)
                        }
                        frame True {
                          n247 = Multiply(x=w558, y=i16 10) -> (x*y=→"Delay 1.6 (B to A)":i16)
                        }
                      }
                      n248 = case shown="True" w348 {
                        tunnel: w220 -> [w552 w553]
                        tunnel: [w551 w553] -> w204
                        frame False {
                          n249 = Increment(x=w552) -> (x+1=w551:i16)
                        }
                        frame True {
                          n250 = Multiply(x=w553, y=i16 10) -> (x*y=→"Delay 1.7 (B to A)":i16)
                        }
                      }
                      n251 = case shown="True" w304 {
                        tunnel: w219 -> [w532 w533]
                        tunnel: [w531 w533] -> w203
                        frame False {
                          n252 = Increment(x=w532) -> (x+1=w531:i16)
                        }
                        frame True {
                          n253 = Multiply(x=w533, y=i16 10) -> (x*y=→"Delay 2.0 (B to A)":i16)
                        }
                      }
                      n254 = case shown="True" w303 {
                        tunnel: w218 -> [w527 w529]
                        tunnel: [w526 w529] -> w202
                        frame False {
                          n255 = Increment(x=w527) -> (x+1=w526:i16)
                        }
                        frame True {
                          n256 = Multiply(x=w529, y=i16 10) -> (x*y=→"Delay 2.1 (B to A)":i16)
                        }
                      }
                      n257 = case shown="True" w292 {
                        tunnel: w215 -> [w512 w514]
                        tunnel: [w511 w514] -> w199
                        frame False {
                          n258 = Increment(x=w512) -> (x+1=w511:i16)
                        }
                        frame True {
                          n259 = Multiply(x=w514, y=i16 10) -> (x*y=→"Delay 2.4 (B to A)":i16)
                        }
                      }
                      n260 = case shown="True" w298 {
                        tunnel: w217 -> [w522 w523]
                        tunnel: [w521 w523] -> w201
                        frame False {
                          n261 = Increment(x=w522) -> (x+1=w521:i16)
                        }
                        frame True {
                          n262 = Multiply(x=w523, y=i16 10) -> (x*y=→"Delay 2.2 (B to A)":i16)
                        }
                      }
                      n263 = case shown="True" w291 {
                        tunnel: w214 -> [w507 w509]
                        tunnel: [w506 w509] -> w198
                        frame False {
                          n264 = Increment(x=w507) -> (x+1=w506:i16)
                        }
                        frame True {
                          n265 = Multiply(x=w509, y=i16 10) -> (x*y=→"Delay 2.5 (B to A)":i16)
                        }
                      }
                      n266 = case shown="True" w297 {
                        tunnel: w216 -> [w517 w519]
                        tunnel: [w516 w519] -> w200
                        frame False {
                          n267 = Increment(x=w517) -> (x+1=w516:i16)
                        }
                        frame True {
                          n268 = Multiply(x=w519, y=i16 10) -> (x*y=→"Delay 2.3 (B to A)":i16)
                        }
                      }
                      n269 = case shown="True" w286 {
                        tunnel: w213 -> [w502 w504]
                        tunnel: [w501 w504] -> w197
                        frame False {
                          n270 = Increment(x=w502) -> (x+1=w501:i16)
                        }
                        frame True {
                          n271 = Multiply(x=w504, y=i16 10) -> (x*y=→"Delay 2.6 (B to A)":i16)
                        }
                      }
                      n272 = case shown="True" w285 {
                        tunnel: w212 -> [w497 w499]
                        tunnel: [w496 w499] -> w196
                        frame False {
                          n273 = Increment(x=w497) -> (x+1=w496:i16)
                        }
                        frame True {
                          n274 = Multiply(x=w499, y=i16 10) -> (x*y=→"Delay 2.7 (B to A)":i16)
                        }
                      }
                      n275 = Boolean To (0,1)(Boolean=w269) -> (0, 1=w267:i16)
                      n276 = Boolean To (0,1)(Boolean=w270) -> (0, 1=w264:i16)
                      n277 = Boolean To (0,1)(Boolean=w271) -> (0, 1=w268:i16)
                      n278 = Equal?(x=w260, y=w273) -> (x = y?=w258:bool)
                      n279 = Equal?(x=w260, y=w274) -> (x = y?=w259:bool)
                      n280 = Scale By Power Of 2(n=i16 1, x=w267) -> (x*2^n=w265:i16)
                      n281 = Scale By Power Of 2(n=i16 2, x=w264) -> (x*2^n=w262:i16)
                      n282 = Compound Arithmetic op=unknown(w268, w265, w262) -> (w261:i16)
                      n283 = local read "Write to PFI"() -> (w251:u8)
                      n284 = To Unsigned Byte Integer(number=w261) -> (unsigned 8bit integer=w252:u8)
                      n285 = Equal?(x=w260, y=w272) -> (x = y?=w257:bool)
                      n286 = local read "Counter"() -> (w351:i16)
                      n287 = Equal?(x=w252, y=w251) -> (x = y?=w256:bool)
                      n288 = Compound Arithmetic op=AND(w259, w258, w257, w256) -> (w255:bool)
                      n289 = Equal?(x=w195, y=w351) -> (x = y?=w254:bool)
                      n290 = Or(x=w255, y=w254) -> (x .or. y?=w253:bool)
                      n291 = case shown="False" w253 {
                        tunnel: [i16 2 i16 1] -> w495
                        tunnel: [FALSE TRUE] -> w494
                        tunnel: w195 -> [w632 w635]
                        tunnel: [w631 w635] -> w249
                        frame False {
                          n292 = Increment(x=w632) -> (x+1=w631:i16)
                        }
                        frame True {
                          "Delay B to A" <- w635
                        }
                      }
                      "Number (B to A)" <- w195
                    }
                    frame 1 {
                      n293 = Number To Boolean Array(number=w639) -> (Boolean array=w673:bool[])
                      n294 = Index Array(array=w673, index=0) -> (element=w674:bool)
                      n295 = Index Array(array=w673, index=2) -> (element=w668:bool)
                      n296 = Index Array(array=w673, index=1) -> (element=w669:bool)
                      n297 = xnode "FPGA I/O Node"("IO Module\\DDCB_Port0_Write"=w638, "IO Module\\DDCB_Port1_Write"=w638, "IO Module\\DDCB_Port2_Write"=w638, "IO Module\\DDCB_PFI1_Write"=w674, "IO Module\\DDCB_PFI2_Write"=w669, "IO Module\\DDCB_PFI3_Write"=w668) -> ()  [unwired: 6 in, 6 out]
                    }
                  }
                }
                frame True {
                  n298 = case shown="2" w738 {
                    tunnel: [i16 1 w1071 i16 2] -> w737
                    tunnel: [FALSE w1070 FALSE] -> w736
                    tunnel: [w768 w825 w1243] -> w735
                    tunnel: w734 -> [w768 w771 w1243]
                    tunnel: w733 -> [_ _ _]
                    tunnel: w678 -> [_ w1069 w1215]
                    tunnel: w678 -> [_ w1059 _]
                    tunnel: [w765 w826 w1242] -> w732
                    tunnel: w731 -> [w765 w824 w1242]
                    tunnel: w730 -> [w764 w823 w1241]
                    tunnel: [w764 w822 w1241] -> w729
                    tunnel: w728 -> [w763 w821 w1240]
                    tunnel: [w763 w820 w1240] -> w727
                    tunnel: w726 -> [w762 w819 w1239]
                    tunnel: w725 -> [w761 w818 w1238]
                    tunnel: w724 -> [w760 w817 w1237]
                    tunnel: w723 -> [w759 w816 w1236]
                    tunnel: w722 -> [w758 w815 w1235]
                    tunnel: [w762 w814 w1239] -> w721
                    tunnel: [w761 w813 w1238] -> w720
                    tunnel: [w760 w812 w1237] -> w719
                    tunnel: [w759 w811 w1236] -> w718
                    tunnel: [w758 w810 w1235] -> w717
                    tunnel: w716 -> [w743 w809 w1216]
                    tunnel: w715 -> [w744 w808 w1217]
                    tunnel: w714 -> [w745 w807 w1218]
                    tunnel: [w745 w806 w1218] -> w713
                    tunnel: [w744 w805 w1217] -> w712
                    tunnel: [w743 w804 w1216] -> w711
                    tunnel: w710 -> [w757 w803 w1234]
                    tunnel: w709 -> [w756 w802 w1233]
                    tunnel: w708 -> [w755 w801 w1232]
                    tunnel: w707 -> [w754 w800 w1231]
                    tunnel: w706 -> [w753 w799 w1230]
                    tunnel: w705 -> [w752 w798 w1229]
                    tunnel: w704 -> [w751 w797 w1228]
                    tunnel: w703 -> [w750 w796 w1227]
                    tunnel: w702 -> [w747 w795 w1224]
                    tunnel: w701 -> [w749 w794 w1226]
                    tunnel: w700 -> [w748 w793 w1225]
                    tunnel: w699 -> [w746 w792 w1223]
                    tunnel: w698 -> [w742 w791 w1222]
                    tunnel: w697 -> [w741 w790 w1221]
                    tunnel: w696 -> [w740 w789 w1220]
                    tunnel: w695 -> [w739 w788 w1219]
                    tunnel: [w757 w787 w1234] -> w694
                    tunnel: [w756 w786 w1233] -> w693
                    tunnel: [w755 w785 w1232] -> w692
                    tunnel: [w754 w784 w1231] -> w691
                    tunnel: [w753 w783 w1230] -> w690
                    tunnel: [w752 w782 w1229] -> w689
                    tunnel: [w751 w781 w1228] -> w688
                    tunnel: [w750 w780 w1227] -> w687
                    tunnel: [w749 w779 w1226] -> w686
                    tunnel: [w748 w778 w1225] -> w685
                    tunnel: [w747 w777 w1224] -> w684
                    tunnel: [w746 w776 w1223] -> w683
                    tunnel: [w742 w775 w1222] -> w682
                    tunnel: [w741 w774 w1221] -> w681
                    tunnel: [w740 w773 w1220] -> w680
                    tunnel: [w739 w772 w1219] -> w679
                    tunnel: w677 -> [_ _ w1214]
                    frame 0, Default {
                      w766 = FALSE ("IO Module\\DDCB_Port0_WE")
                      w770 = TRUE
                      n299 = xnode "FPGA I/O Node"("IO Module\\DDCA_Port0_WE"=w770, "IO Module\\DDCA_Port1_WE"=w770, "IO Module\\DDCA_Port2_WE"=w770, "IO Module\\DDCA_PFI_WE"=w770, "IO Module\\DDCB_Port0_WE"=w766, "IO Module\\DDCB_Port1_WE"=w766, "IO Module\\DDCB_Port2_WE"=w766, "IO Module\\DDCB_PFI_WE"=w766) -> ()  [unwired: 8 in, 8 out]
                    }
                    frame 2 {
                      # "Write to"
                      # "PFI"
                      n300 = xnode "FPGA I/O Node"() -> ("IO Module\\DDCB_Port0_Read"=w1045:u8, "IO Module\\DDCB_Port1_Read"=w1035:u8, "IO Module\\DDCB_Port2_Read"=w1025:u8, "IO Module\\DDCB_PFI1_Read"=w962:bool, "IO Module\\DDCB_PFI2_Read"=w961:bool, "IO Module\\DDCB_PFI3_Read"=w960:bool)  [unwired: 6 in, 6 out]
                      n301 = Number To Boolean Array(number=w1059) -> (Boolean array=w1055:bool[])
                      n302 = Number To Boolean Array(number=w1069) -> (Boolean array=w1068:bool[])
                      n303 = Index Array(array=w1068, index=5) -> (element=→"5":bool)
                      n304 = Index Array(array=w1068, index=7) -> (element=→"7":bool)
                      n305 = Index Array(array=w1068, index=4) -> (element=→"4":bool)
                      n306 = Index Array(array=w1068, index=6) -> (element=→"6":bool)
                      n307 = Index Array(array=w1068, index=2) -> (element=→"2":bool)
                      n308 = Index Array(array=w1068, index=3) -> (element=→"3":bool)
                      n309 = Index Array(array=w1055, index=2) -> (element=→"PFI 3  (A to B)":bool)
                      n310 = Index Array(array=w1068, index=1) -> (element=→"1":bool)
                      n311 = Index Array(array=w1055, index=1) -> (element=→"PFI 2  (A to B)":bool)
                      n312 = Index Array(array=w1068, index=0) -> (element=→"0":bool)
                      n313 = Index Array(array=w1055, index=0) -> (element=→"PFI 1  (A to B)":bool)
                      n314 = Number To Boolean Array(number=w1025) -> (Boolean array=w1026:bool[])
                      n315 = Number To Boolean Array(number=w1035) -> (Boolean array=w1044:bool[])
                      n316 = Number To Boolean Array(number=w1045) -> (Boolean array=w1046:bool[])
                      n317 = local read "PFI 1  (A to B)"() -> (w965:bool)
                      n318 = local read "PFI 2  (A to B)"() -> (w964:bool)
                      n319 = local read "PFI 3  (A to B)"() -> (w963:bool)
                      n320 = Index Array(array=w1026, index=5) -> (element=w968:bool)
                      n321 = Index Array(array=w1026, index=7) -> (element=w966:bool)
                      n322 = Index Array(array=w1026, index=4) -> (element=w969:bool)
                      n323 = Index Array(array=w1026, index=6) -> (element=w967:bool)
                      n324 = Index Array(array=w1026, index=2) -> (element=w971:bool)
                      n325 = Index Array(array=w1026, index=3) -> (element=w970:bool)
                      n326 = Index Array(array=w1026, index=1) -> (element=w972:bool)
                      n327 = Index Array(array=w1044, index=5) -> (element=w984:bool)
                      n328 = Index Array(array=w1044, index=7) -> (element=w982:bool)
                      n329 = Index Array(array=w1026, index=0) -> (element=w973:bool)
                      n330 = Index Array(array=w1044, index=4) -> (element=w985:bool)
                      n331 = Index Array(array=w1044, index=6) -> (element=w983:bool)
                      n332 = Index Array(array=w1044, index=2) -> (element=w987:bool)
                      n333 = Index Array(array=w1044, index=3) -> (element=w986:bool)
                      n334 = Index Array(array=w1044, index=1) -> (element=w988:bool)
                      n335 = Index Array(array=w1046, index=5) -> (element=w1002:bool)
                      n336 = Index Array(array=w1046, index=7) -> (element=w998:bool)
                      n337 = Index Array(array=w1044, index=0) -> (element=w989:bool)
                      n338 = Index Array(array=w1046, index=4) -> (element=w1004:bool)
                      n339 = Index Array(array=w1046, index=6) -> (element=w1000:bool)
                      n340 = Index Array(array=w1046, index=2) -> (element=w1008:bool)
                      n341 = Index Array(array=w1046, index=3) -> (element=w1006:bool)
                      n342 = Index Array(array=w1046, index=1) -> (element=w1010:bool)
                      n343 = Index Array(array=w1046, index=0) -> (element=w1013:bool)
                      n344 = local read "7"() -> (w999:bool)
                      n345 = local read "6"() -> (w1001:bool)
                      n346 = local read "3"() -> (w1007:bool)
                      n347 = local read "5"() -> (w1003:bool)
                      n348 = local read "7"() -> (w997:bool)
                      n349 = local read "6"() -> (w996:bool)
                      n350 = local read "7"() -> (w974:bool)
                      n351 = local read "2"() -> (w1009:bool)
                      n352 = local read "4"() -> (w1005:bool)
                      n353 = local read "3"() -> (w993:bool)
                      n354 = local read "5"() -> (w995:bool)
                      n355 = local read "6"() -> (w975:bool)
                      n356 = local read "2"() -> (w992:bool)
                      n357 = local read "4"() -> (w994:bool)
                      n358 = local read "3"() -> (w978:bool)
                      n359 = local read "5"() -> (w976:bool)
                      n360 = local read "0"() -> (w1012:bool)
                      n361 = local read "1"() -> (w1011:bool)
                      n362 = local read "2"() -> (w979:bool)
                      n363 = local read "4"() -> (w977:bool)
                      n364 = local read "0"() -> (w990:bool)
                      n365 = local read "1"() -> (w991:bool)
                      n366 = local read "0"() -> (w981:bool)
                      n367 = local read "1"() -> (w980:bool)
                      n368 = Equal?(x=w965, y=w962) -> (x = y?=w885:bool)
                      n369 = Equal?(x=w964, y=w961) -> (x = y?=w884:bool)
                      n370 = Equal?(x=w1001, y=w1000) -> (x = y?=w929:bool)
                      n371 = Equal?(x=w999, y=w998) -> (x = y?=w928:bool)
                      n372 = Equal?(x=w990, y=w989) -> (x = y?=w902:bool)
                      n373 = Equal?(x=w963, y=w960) -> (x = y?=w883:bool)
                      n374 = Equal?(x=w991, y=w988) -> (x = y?=w901:bool)
                      n375 = Equal?(x=w996, y=w983) -> (x = y?=w896:bool)
                      n376 = Equal?(x=w997, y=w982) -> (x = y?=w895:bool)
                      n377 = Equal?(x=w1005, y=w1004) -> (x = y?=w940:bool)
                      n378 = Equal?(x=w1003, y=w1002) -> (x = y?=w930:bool)
                      n379 = Equal?(x=w992, y=w987) -> (x = y?=w900:bool)
                      n380 = Equal?(x=w974, y=w966) -> (x = y?=w851:bool)
                      n381 = Equal?(x=w1009, y=w1008) -> (x = y?=w948:bool)
                      n382 = Equal?(x=w1007, y=w1006) -> (x = y?=w944:bool)
                      n383 = Equal?(x=w993, y=w986) -> (x = y?=w899:bool)
                      n384 = Equal?(x=w975, y=w967) -> (x = y?=w852:bool)
                      n385 = Equal?(x=w994, y=w985) -> (x = y?=w898:bool)
                      n386 = Equal?(x=w995, y=w984) -> (x = y?=w897:bool)
                      n387 = Equal?(x=w1012, y=w1013) -> (x = y?=w959:bool)
                      n388 = Equal?(x=w1011, y=w1010) -> (x = y?=w952:bool)
                      n389 = Equal?(x=w977, y=w969) -> (x = y?=w854:bool)
                      n390 = Equal?(x=w976, y=w968) -> (x = y?=w853:bool)
                      n391 = Equal?(x=w979, y=w971) -> (x = y?=w856:bool)
                      n392 = Equal?(x=w978, y=w970) -> (x = y?=w855:bool)
                      n393 = Equal?(x=w981, y=w973) -> (x = y?=w858:bool)
                      n394 = Equal?(x=w980, y=w972) -> (x = y?=w857:bool)
                      n395 = local read "Counter"() -> (w892:i16)
                      n396 = local read "Counter"() -> (w891:i16)
                      n397 = local read "Counter"() -> (w886:i16)
                      n398 = local read "Counter"() -> (w958:i16)
                      n399 = local read "Counter"() -> (w953:i16)
                      n400 = local read "Counter"() -> (w951:i16)
                      n401 = local read "Counter"() -> (w945:i16)
                      n402 = local read "Counter"() -> (w943:i16)
                      n403 = local read "Counter"() -> (w937:i16)
                      n404 = local read "Counter"() -> (w936:i16)
                      n405 = local read "Counter"() -> (w931:i16)
                      n406 = xnode "FPGA I/O Node"() -> ("IO Module\\DDCB_Port0_Read"=w850:u8, "IO Module\\DDCB_Port1_Read"=w849:u8, "IO Module\\DDCB_Port2_Read"=w848:u8, "IO Module\\DDCB_PFI1_Read"=w847:bool, "IO Module\\DDCB_PFI2_Read"=w845:bool, "IO Module\\DDCB_PFI3_Read"=w846:bool)  [unwired: 6 in, 6 out]
                      "Read Port 0 B" <- w850
                      "Read Port 1 B" <- w849
                      "Read Port 2 B" <- w848
                      "DDCB_PFI1_Read (A to B)" <- w847
                      "DDCB_PFI2_Read (A to B)" <- w845
                      "DDCB_PFI3_Read (A to B)" <- w846
                      n407 = Equal?(x=w809, y=w892) -> (x = y?=w893:bool)
                      n408 = Equal?(x=w808, y=w891) -> (x = y?=w890:bool)
                      n409 = Equal?(x=w807, y=w886) -> (x = y?=w887:bool)
                      n410 = local read "Counter"() -> (w903:i16)
                      n411 = local read "Counter"() -> (w908:i16)
                      n412 = local read "Counter"() -> (w909:i16)
                      n413 = local read "Counter"() -> (w914:i16)
                      n414 = local read "Counter"() -> (w915:i16)
                      n415 = local read "Counter"() -> (w920:i16)
                      n416 = local read "Counter"() -> (w921:i16)
                      n417 = local read "Counter"() -> (w926:i16)
                      n418 = local read "Counter"() -> (w882:i16)
                      n419 = local read "Counter"() -> (w877:i16)
                      n420 = local read "Counter"() -> (w876:i16)
                      n421 = Equal?(x=w824, y=w958) -> (x = y?=w957:bool)
                      n422 = local read "Counter"() -> (w871:i16)
                      n423 = Or(x=w885, y=w893) -> (x .or. y?=w894:bool)
                      n424 = Or(x=w884, y=w890) -> (x .or. y?=w889:bool)
                      n425 = Or(x=w883, y=w887) -> (x .or. y?=w888:bool)
                      n426 = local read "Counter"() -> (w870:i16)
                      n427 = Equal?(x=w823, y=w953) -> (x = y?=w954:bool)
                      n428 = local read "Counter"() -> (w865:i16)
                      n429 = local read "Counter"() -> (w864:i16)
                      n430 = local read "Counter"() -> (w859:i16)
                      n431 = Equal?(x=w821, y=w951) -> (x = y?=w950:bool)
                      n432 = Equal?(x=w819, y=w945) -> (x = y?=w946:bool)
                      n433 = Equal?(x=w818, y=w943) -> (x = y?=w942:bool)
                      n434 = Equal?(x=w817, y=w937) -> (x = y?=w938:bool)
                      n435 = Equal?(x=w816, y=w936) -> (x = y?=w935:bool)
                      n436 = Equal?(x=w815, y=w931) -> (x = y?=w932:bool)
                      n437 = case shown="True" w894 {
                        tunnel: w809 -> [w1123 w1124]
                        tunnel: [w1122 w1124] -> w804
                        frame False {
                          n438 = Increment(x=w1123) -> (x+1=w1122:i16)
                        }
                        frame True {
                          n439 = Multiply(x=w1124, y=i16 10) -> (x*y=→"Delay PFI1":i16)
                        }
                      }
                      n440 = case shown="True" w889 {
                        tunnel: w808 -> [w1118 w1119]
                        tunnel: [w1117 w1119] -> w805
                        frame False {
                          n441 = Increment(x=w1118) -> (x+1=w1117:i16)
                        }
                        frame True {
                          n442 = Multiply(x=w1119, y=i16 10) -> (x*y=→"Delay PFI2":i16)
                        }
                      }
                      n443 = case shown="True" w888 {
                        tunnel: w807 -> [w1113 w1114]
                        tunnel: [w1112 w1114] -> w806
                        frame False {
                          n444 = Increment(x=w1113) -> (x+1=w1112:i16)
                        }
                        frame True {
                          n445 = Multiply(x=w1114, y=i16 10) -> (x*y=→"Delay PFI3":i16)
                        }
                      }
                      n446 = Or(x=w959, y=w957) -> (x .or. y?=w956:bool)
                      n447 = Or(x=w952, y=w954) -> (x .or. y?=w955:bool)
                      n448 = Or(x=w948, y=w950) -> (x .or. y?=w949:bool)
                      n449 = Or(x=w944, y=w946) -> (x .or. y?=w947:bool)
                      n450 = Equal?(x=w803, y=w903) -> (x = y?=w904:bool)
                      n451 = Or(x=w940, y=w942) -> (x .or. y?=w941:bool)
                      n452 = Or(x=w930, y=w938) -> (x .or. y?=w939:bool)
                      n453 = Equal?(x=w802, y=w908) -> (x = y?=w907:bool)
                      n454 = Or(x=w929, y=w935) -> (x .or. y?=w934:bool)
                      n455 = Or(x=w928, y=w932) -> (x .or. y?=w933:bool)
                      n456 = Equal?(x=w801, y=w909) -> (x = y?=w910:bool)
                      n457 = Equal?(x=w800, y=w914) -> (x = y?=w913:bool)
                      n458 = Equal?(x=w799, y=w915) -> (x = y?=w916:bool)
                      n459 = Equal?(x=w798, y=w920) -> (x = y?=w919:bool)
                      n460 = Equal?(x=w797, y=w921) -> (x = y?=w922:bool)
                      n461 = Equal?(x=w796, y=w926) -> (x = y?=w925:bool)
                      n462 = Equal?(x=w795, y=w882) -> (x = y?=w881:bool)
                      n463 = case shown="True" w956 {
                        tunnel: w824 -> [w1202 w1204]
                        tunnel: [w1203 w1204] -> w826
                        frame False {
                          n464 = Increment(x=w1202) -> (x+1=w1203:i16)
                        }
                        frame True {
                          n465 = Multiply(x=w1204, y=i16 10) -> (x*y=→"Delay 0.0":i16)
                        }
                      }
                      n466 = Equal?(x=w794, y=w877) -> (x = y?=w878:bool)
                      n467 = Equal?(x=w793, y=w876) -> (x = y?=w875:bool)
                      n468 = Equal?(x=w792, y=w871) -> (x = y?=w872:bool)
                      n469 = case shown="True" w955 {
                        tunnel: w823 -> [w1198 w1199]
                        tunnel: [w1197 w1199] -> w822
                        frame False {
                          n470 = Increment(x=w1198) -> (x+1=w1197:i16)
                        }
                        frame True {
                          n471 = Multiply(x=w1199, y=i16 10) -> (x*y=→"Delay 0.1":i16)
                        }
                      }
                      n472 = case shown="True" w941 {
                        tunnel: w818 -> [w1183 w1184]
                        tunnel: [w1182 w1184] -> w813
                        frame False {
                          n473 = Increment(x=w1183) -> (x+1=w1182:i16)
                        }
                        frame True {
                          n474 = Multiply(x=w1184, y=i16 10) -> (x*y=→"Delay 0.4":i16)
                        }
                      }
                      n475 = Equal?(x=w791, y=w870) -> (x = y?=w869:bool)
                      n476 = case shown="True" w949 {
                        tunnel: w821 -> [w1193 w1194]
                        tunnel: [w1192 w1194] -> w820
                        frame False {
                          n477 = Increment(x=w1193) -> (x+1=w1192:i16)
                        }
                        frame True {
                          n478 = Multiply(x=w1194, y=i16 10) -> (x*y=→"Delay 0.2":i16)
                        }
                      }
                      n479 = Or(x=w902, y=w904) -> (x .or. y?=w905:bool)
                      n480 = case shown="True" w939 {
                        tunnel: w817 -> [w1178 w1180]
                        tunnel: [w1177 w1180] -> w812
                        frame False {
                          n481 = Increment(x=w1178) -> (x+1=w1177:i16)
                        }
                        frame True {
                          n482 = Multiply(x=w1180, y=i16 10) -> (x*y=→"Delay 0.5":i16)
                        }
                      }
                      n483 = case shown="True" w947 {
                        tunnel: w819 -> [w1188 w1189]
                        tunnel: [w1187 w1189] -> w814
                        frame False {
                          n484 = Increment(x=w1188) -> (x+1=w1187:i16)
                        }
                        frame True {
                          n485 = Multiply(x=w1189, y=i16 10) -> (x*y=→"Delay 0.3":i16)
                        }
                      }
                      n486 = case shown="True" w934 {
                        tunnel: w816 -> [w1173 w1174]
                        tunnel: [w1172 w1174] -> w811
                        frame False {
                          n487 = Increment(x=w1173) -> (x+1=w1172:i16)
                        }
                        frame True {
                          n488 = Multiply(x=w1174, y=i16 10) -> (x*y=→"Delay 0.6":i16)
                        }
                      }
                      n489 = case shown="True" w933 {
                        tunnel: w815 -> [w1168 w1170]
                        tunnel: [w1167 w1170] -> w810
                        frame False {
                          n490 = Increment(x=w1168) -> (x+1=w1167:i16)
                        }
                        frame True {
                          n491 = Multiply(x=w1170, y=i16 10) -> (x*y=→"Delay 0.7":i16)
                        }
                      }
                      n492 = Equal?(x=w790, y=w865) -> (x = y?=w866:bool)
                      n493 = Equal?(x=w789, y=w864) -> (x = y?=w863:bool)
                      n494 = Equal?(x=w788, y=w859) -> (x = y?=w860:bool)
                      n495 = Or(x=w901, y=w907) -> (x .or. y?=w906:bool)
                      n496 = Or(x=w900, y=w910) -> (x .or. y?=w911:bool)
                      n497 = Or(x=w899, y=w913) -> (x .or. y?=w912:bool)
                      n498 = Or(x=w898, y=w916) -> (x .or. y?=w917:bool)
                      n499 = Or(x=w897, y=w919) -> (x .or. y?=w918:bool)
                      n500 = Or(x=w896, y=w922) -> (x .or. y?=w923:bool)
                      n501 = Or(x=w895, y=w925) -> (x .or. y?=w924:bool)
                      n502 = Or(x=w858, y=w881) -> (x .or. y?=w880:bool)
                      n503 = Or(x=w857, y=w878) -> (x .or. y?=w879:bool)
                      n504 = Or(x=w856, y=w875) -> (x .or. y?=w874:bool)
                      n505 = Or(x=w855, y=w872) -> (x .or. y?=w873:bool)
                      n506 = Or(x=w854, y=w869) -> (x .or. y?=w868:bool)
                      n507 = case shown="True" w905 {
                        tunnel: w803 -> [w1163 w1165]
                        tunnel: [w1162 w1165] -> w787
                        frame False {
                          n508 = Increment(x=w1163) -> (x+1=w1162:i16)
                        }
                        frame True {
                          n509 = Multiply(x=w1165, y=i16 10) -> (x*y=→"Delay 1.0":i16)
                        }
                      }
                      n510 = Or(x=w853, y=w866) -> (x .or. y?=w867:bool)
                      n511 = Or(x=w852, y=w863) -> (x .or. y?=w862:bool)
                      n512 = Or(x=w851, y=w860) -> (x .or. y?=w861:bool)
                      n513 = local read "Write to"() -> (w836:u8)
                      n514 = case shown="True" w906 {
                        tunnel: w802 -> [w1158 w1160]
                        tunnel: [w1157 w1160] -> w786
                        frame False {
                          n515 = Increment(x=w1158) -> (x+1=w1157:i16)
                        }
                        frame True {
                          n516 = Multiply(x=w1160, y=i16 10) -> (x*y=→"Delay 1.1":i16)
                        }
                      }
                      n517 = case shown="True" w917 {
                        tunnel: w799 -> [w1143 w1145]
                        tunnel: [w1142 w1145] -> w783
                        frame False {
                          n518 = Increment(x=w1143) -> (x+1=w1142:i16)
                        }
                        frame True {
                          n519 = Multiply(x=w1145, y=i16 10) -> (x*y=→"Delay 1.4":i16)
                        }
                      }
                      n520 = case shown="True" w911 {
                        tunnel: w801 -> [w1153 w1155]
                        tunnel: [w1152 w1155] -> w785
                        frame False {
                          n521 = Increment(x=w1153) -> (x+1=w1152:i16)
                        }
                        frame True {
                          n522 = Multiply(x=w1155, y=i16 10) -> (x*y=→"Delay 1.2":i16)
                        }
                      }
                      n523 = case shown="True" w918 {
                        tunnel: w798 -> [w1138 w1140]
                        tunnel: [w1137 w1140] -> w782
                        frame False {
                          n524 = Increment(x=w1138) -> (x+1=w1137:i16)
                        }
                        frame True {
                          n525 = Multiply(x=w1140, y=i16 10) -> (x*y=→"Delay 1.5":i16)
                        }
                      }
                      n526 = case shown="True" w912 {
                        tunnel: w800 -> [w1148 w1149]
                        tunnel: [w1147 w1149] -> w784
                        frame False {
                          n527 = Increment(x=w1148) -> (x+1=w1147:i16)
                        }
                        frame True {
                          n528 = Multiply(x=w1149, y=i16 10) -> (x*y=→"Delay 1.3":i16)
                        }
                      }
                      n529 = case shown="True" w923 {
                        tunnel: w797 -> [w1133 w1134]
                        tunnel: [w1132 w1134] -> w781
                        frame False {
                          n530 = Increment(x=w1133) -> (x+1=w1132:i16)
                        }
                        frame True {
                          n531 = Multiply(x=w1134, y=i16 10) -> (x*y=→"Delay 1.6":i16)
                        }
                      }
                      n532 = case shown="True" w924 {
                        tunnel: w796 -> [w1128 w1129]
                        tunnel: [w1127 w1129] -> w780
                        frame False {
                          n533 = Increment(x=w1128) -> (x+1=w1127:i16)
                        }
                        frame True {
                          n534 = Multiply(x=w1129, y=i16 10) -> (x*y=→"Delay 1.7":i16)
                        }
                      }
                      n535 = case shown="True" w880 {
                        tunnel: w795 -> [w1108 w1109]
                        tunnel: [w1107 w1109] -> w779
                        frame False {
                          n536 = Increment(x=w1108) -> (x+1=w1107:i16)
                        }
                        frame True {
                          n537 = Multiply(x=w1109, y=i16 10) -> (x*y=→"Delay 2.0":i16)
                        }
                      }
                      n538 = case shown="True" w879 {
                        tunnel: w794 -> [w1103 w1105]
                        tunnel: [w1102 w1105] -> w778
                        frame False {
                          n539 = Increment(x=w1103) -> (x+1=w1102:i16)
                        }
                        frame True {
                          n540 = Multiply(x=w1105, y=i16 10) -> (x*y=→"Delay 2.1":i16)
                        }
                      }
                      n541 = case shown="True" w868 {
                        tunnel: w791 -> [w1088 w1089]
                        tunnel: [w1087 w1089] -> w775
                        frame False {
                          n542 = Increment(x=w1088) -> (x+1=w1087:i16)
                        }
                        frame True {
                          n543 = Multiply(x=w1089, y=i16 10) -> (x*y=→"Delay 2.4":i16)
                        }
                      }
                      n544 = case shown="True" w874 {
                        tunnel: w793 -> [w1098 w1100]
                        tunnel: [w1097 w1100] -> w777
                        frame False {
                          n545 = Increment(x=w1098) -> (x+1=w1097:i16)
                        }
                        frame True {
                          n546 = Multiply(x=w1100, y=i16 10) -> (x*y=→"Delay 2.2":i16)
                        }
                      }
                      n547 = case shown="True" w867 {
                        tunnel: w790 -> [w1083 w1084]
                        tunnel: [w1082 w1084] -> w774
                        frame False {
                          n548 = Increment(x=w1083) -> (x+1=w1082:i16)
                        }
                        frame True {
                          n549 = Multiply(x=w1084, y=i16 10) -> (x*y=→"Delay 2.5":i16)
                        }
                      }
                      n550 = case shown="True" w873 {
                        tunnel: w792 -> [w1093 w1094]
                        tunnel: [w1092 w1094] -> w776
                        frame False {
                          n551 = Increment(x=w1093) -> (x+1=w1092:i16)
                        }
                        frame True {
                          n552 = Multiply(x=w1094, y=i16 10) -> (x*y=→"Delay 2.3":i16)
                        }
                      }
                      n553 = case shown="True" w862 {
                        tunnel: w789 -> [w1078 w1080]
                        tunnel: [w1077 w1080] -> w773
                        frame False {
                          n554 = Increment(x=w1078) -> (x+1=w1077:i16)
                        }
                        frame True {
                          n555 = Multiply(x=w1080, y=i16 10) -> (x*y=→"Delay 2.6":i16)
                        }
                      }
                      n556 = case shown="True" w861 {
                        tunnel: w788 -> [w1073 w1074]
                        tunnel: [w1072 w1074] -> w772
                        frame False {
                          n557 = Increment(x=w1073) -> (x+1=w1072:i16)
                        }
                        frame True {
                          n558 = Multiply(x=w1074, y=i16 10) -> (x*y=→"Delay 2.7":i16)
                        }
                      }
                      n559 = Boolean To (0,1)(Boolean=w845) -> (0, 1=w843:i16)
                      n560 = Boolean To (0,1)(Boolean=w846) -> (0, 1=w840:i16)
                      n561 = Boolean To (0,1)(Boolean=w847) -> (0, 1=w844:i16)
                      n562 = Equal?(x=w836, y=w849) -> (x = y?=w834:bool)
                      n563 = Equal?(x=w836, y=w850) -> (x = y?=w835:bool)
                      n564 = Scale By Power Of 2(n=i16 1, x=w843) -> (x*2^n=w841:i16)
                      n565 = Scale By Power Of 2(n=i16 2, x=w840) -> (x*2^n=w838:i16)
                      n566 = Compound Arithmetic op=unknown(w844, w841, w838) -> (w837:i16)
                      n567 = local read "Write to PFI"() -> (w827:u8)
                      n568 = To Unsigned Byte Integer(number=w837) -> (unsigned 8bit integer=w828:u8)
                      n569 = Equal?(x=w836, y=w848) -> (x = y?=w833:bool)
                      n570 = local read "Counter"() -> (w927:i16)
                      n571 = Equal?(x=w828, y=w827) -> (x = y?=w832:bool)
                      n572 = Compound Arithmetic op=AND(w835, w834, w833, w832) -> (w831:bool)
                      n573 = Equal?(x=w771, y=w927) -> (x = y?=w830:bool)
                      n574 = Or(x=w831, y=w830) -> (x .or. y?=w829:bool)
                      n575 = case shown="False" w829 {
                        tunnel: [i16 2 i16 1] -> w1071
                        tunnel: [FALSE TRUE] -> w1070
                        tunnel: w771 -> [w1208 w1211]
                        tunnel: [w1207 w1211] -> w825
                        frame False {
                          n576 = Increment(x=w1208) -> (x+1=w1207:i16)
                        }
                        frame True {
                          "Delay A to B" <- w1211
                        }
                      }
                    }
                    frame 1 {
                      n577 = Number To Boolean Array(number=w1215) -> (Boolean array=w1249:bool[])
                      n578 = Index Array(array=w1249, index=0) -> (element=w1250:bool)
                      n579 = Index Array(array=w1249, index=2) -> (element=w1244:bool)
                      n580 = Index Array(array=w1249, index=1) -> (element=w1245:bool)
                      n581 = xnode "FPGA I/O Node"("IO Module\\DDCA_Port0_Write"=w1214, "IO Module\\DDCA_Port1_Write"=w1214, "IO Module\\DDCA_Port2_Write"=w1214, "IO Module\\DDCA_PFI1_Write"=w1250, "IO Module\\DDCA_PFI2_Write"=w1245, "IO Module\\DDCA_PFI3_Write"=w1244) -> ()  [unwired: 6 in, 6 out]
                    }
                  }
                }
              }
            }
            n582 = node-c288(w37) -> ()
          }
          frame #2 {
            n583 = local write "Cycle"(FALSE ("Cycle")) -> ()
            "Operation compl" <- TRUE ("Boolean")
          }
        }
      }
    }
  }
